vi "sub_hw-seq-all.vi"(8 "error":errorcluster, 11 "HWseq":T1) -> (0 "error out":errorcluster)   [LabVIEW 2019]
uses:
  rc-seq_enum.ctl
  SubVIs/common/_ctrl/system-status.ctl
  _ctrl/rw.ctl
  SubVIs/cmd_timer.ctl
  sequence_single.ctl
  SubVIs/common/hw-control.ctl
  common/UI.ctl
  common/cmd_timecheck.ctl
  _ctrl/BP4610_cmd.ctl
  breakdown.ctl
  SubVIs/common/cmd_offtimecheck.ctl
  _ctrl/init-r-stop.ctl
  58aef34a-c39e-4a76-bc91-cdbe2ad7e567.vi
  310223a1-0247-4d5e-a4de-31e905c381c2.vi
  d9d656a3-d7bb-48da-8160-e06b142862e8.vi
  66709171-801d-4df5-8281-070cbfffc908.vi
  b680e723-f219-401b-b6b8-117c4d919767.vi
  acb3f5d6-e9ea-41c1-b59f-33d80ec98a9a.vi
  88b04c44-2d0f-4c5f-adc0-824f85c1baca.vi
  7df0aa0f-9000-4fc8-8be1-235500cee508.vi
  a3ee31cb-2ee6-4b2e-876a-aa05c6fd3f6c.vi
  a1681bb8-cff8-4085-a791-91921f38d214.vi
  0886c58b-0a1e-4b1c-982a-d26cf992a476.vi
  1d089e96-dcf8-4fa6-b139-0f624cb7beb8.vi
  05f56422-7d15-472a-846f-8a5a9856abb2.vi
  7e616775-0fa7-4587-9f3e-cf6cd70ddc46.vi
  c0c5eac8-8ea9-47a8-809d-3af25785a4f7.vi
  9bb39240-68e1-431b-a926-99d42a230205.vi
  e7f2ea11-fc70-48eb-a069-d8d263784f6c.vi
  1f2546c3-2858-4bb2-b627-ba606493a871.vi
  SubVIs/common/Glob_Ref.vi
panel:
  in  "Numeric":i32
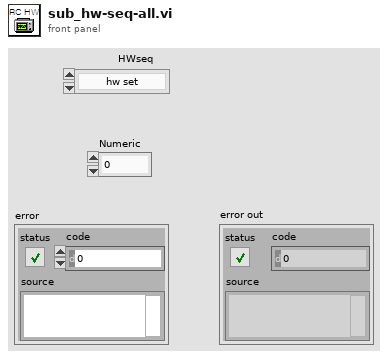
[diagram p1: front panel]
types:
  T1 = typedef "rc-seq_enum.ctl" = enum16{"hw set", "Pwr-in on", "ch-relay on", "Pwr-out on", "AO on", "AO 0v", "Pwr-in off", "Relay-all off", "Pwr-out off", "Discharge", "950 read", "Run", "Stop"}
  T2 = typedef "sequence_single.ctl" = enum16{"Register", "RC", "B1", "B2", "B3", "Oper_LV", "Oper_HV", "ContR_LV"}
  T3 = typedef "cmd_timer.ctl" = enum16{"init", "init_update", "run", "default", "update"}
  T4 = typedef "rw.ctl" = enum16{"read", "write"}
  T5 = typedef "system-status.ctl" = enum16{"Initial", "Update", "Clear", "Read"}
  T6 = typedef "ui_dev-operator.ctl" = cluster{"Operation stutus":refnum<vi>, "Test Status":refnum<vi>, "Setting":refnum<vi>, "Manual":refnum<vi>, "Main":refnum<vi>, "RCstart":refnum<vi>, "채널선택":refnum<vi>, "시험명":refnum<vi>, "Tab Control_manual":refnum<vi>, "시험 모드":refnum<vi>, "HW check":refnum<vi>, "login":refnum<vi>, "logout":refnum<vi>}
  T7 = typedef "Testing-info.ctl" = cluster{"전체채널수":u8, "현재채널번호":u8, "Irms":dbl, "입력전압":dbl, "입력전류":dbl, "출력전압":dbl, "출력전류":dbl, "온도":dbl, "제어단 단선":bool, "제어단 단락":bool, "제어단 특성변화":bool, "출력단 단선":bool, "출력단 단락":bool, "출력단 특성변화":bool, "출력단 전압":bool, "카운트 일치":bool, "Irms 판정":bool, "온도":bool, "테스트 회수":u32, "TestType":T2, "현재회수":u32, "Ch selection":cluster{"1ch":bool, "2ch":bool, "3ch":bool, "4ch":bool, "5ch":bool, "6ch":bool}, "반복":u32, "Path":path, "파일생성주기":u32, "start time":dbl, "stop time":dbl, "현재반복회수":u32, "NG":cluster{"입출력 카운트":bool, "출력전류RMS":bool}}
  T8 = cluster{"1ch":bool, "2ch":bool, "3ch":bool, "4ch":bool, "5ch":bool, "6ch":bool}
  T9 = typedef "hw-control.ctl" = enum16{"DL950 ready", "DL950 clear", "DL950 trigger", "DL950 read", "DL950 read seq", "DL950 Tsingle query", "AO 12v", "AO wave", "AO 0v", "relay all-off", "Discharge check", "Discharge", "Relay1", "Relay2", "Relay3", "Relay4", "Relay5", "Relay6", "BP4610 onoff", "BP4610 set", "DSP1500 set", "DSP1500 onoff"}
  T10 = typedef "UI.ctl" = enum16{"Alarm yellow", "DL950 graph show", "DL950 graph clear", "AO value", "AO blink onoff", "Discharge relay", "Input Power", "Outpower", "Relay in1", "Relay in2", "Relay in3", "Relay in4", "Relay in5", "Relay in6", "Relay out1", "Relay out2", "Relay out3", "Relay out4", "Relay out5", "Relay out6", "Relay all off"}
  T11 = typedef "cmd_timecheck.ctl" = enum16{"Group start", "Group end", "Grout dt", "Ch start", "Ch end", "Ch dt", "init", "NF start", "NF stop", "idrc start", "idrc stop", "scope start", "scope stop", "ao start", "ao stop", "relay start", "relay stop", "NF read start", "NF read stop", "NF set start", "NF set stop", "idrc level start", "idrc level stop", "scope trig start", "scope trig stop", "relay dischar star", "relay dischar stop", "data process start", "data process stop", "ch-relay on start", "ch-relay on stop", "hw set start", "hw set stop", "pwr-in on start", "pwr-in on stop", "pwr-out on start", "pwr-out on stop", "ao on start", "ao on stop", "ao 0v start", "ao 0v stop", "pwr-in off start", "pwr-in off stop", "relay-all off start", "relay-all off stop", "pwr-out off start", "pwr-out off stop", "discharge start", "discharge stop", "950 read start", "950 read stop"}
  T12 = typedef "BP4610_cmd.ctl" = enum16{"open", "read", "set", "set_seq", "limit", "limit_seq", "output on", "output off", "close"}
  T13 = typedef "breakdown.ctl" = enum16{"DL950 items", "input pwr", "output pwr", "output pwr_adv"}
  T14 = typedef "cmd_offtimecheck.ctl" = enum16{"start", "check", "init"}
  T15 = typedef "Error list.ctl" = cluster{"DL950":bool, "BP4610":bool, "DSP":bool, "AI":bool, "AO":bool, "DO":bool}
  T16 = typedef "init-r-stop.ctl" = enum16{"ini", "read", "stop"}
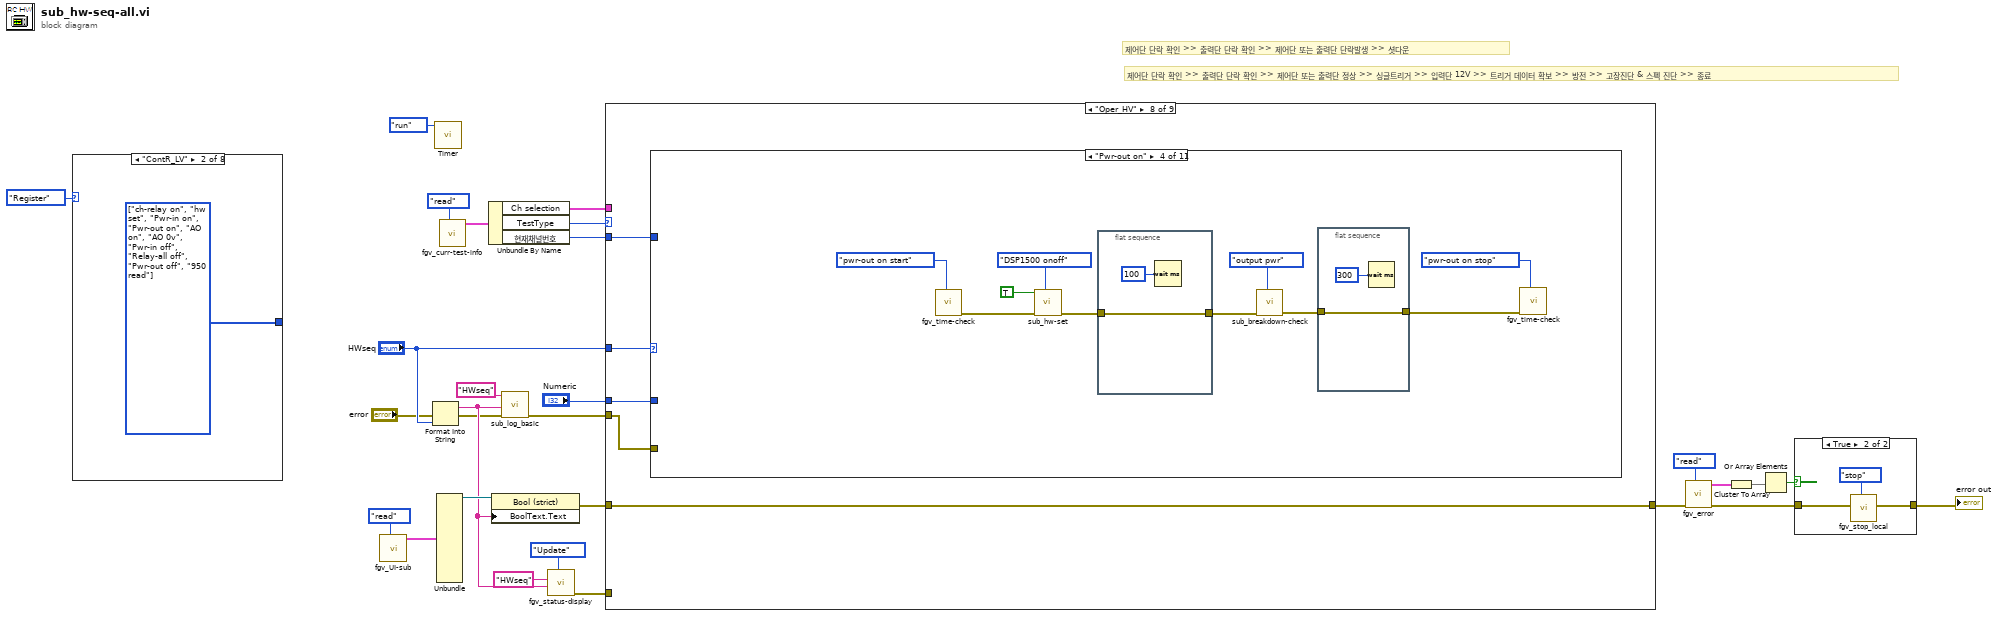
[diagram p0: block diagram]
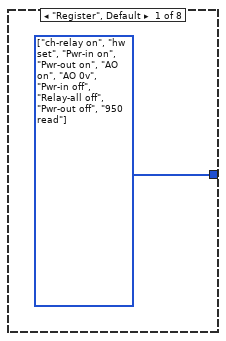
[diagram p2: hidden frame]
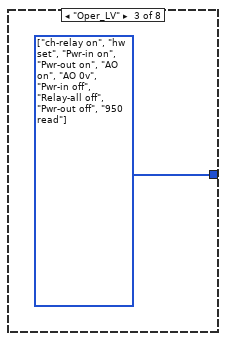
[diagram p3: hidden frame]
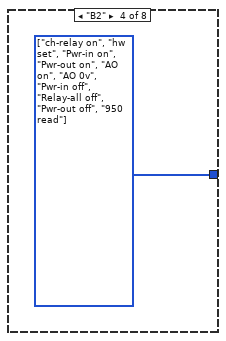
[diagram p4: hidden frame]
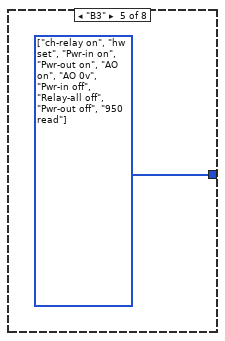
[diagram p5: hidden frame]
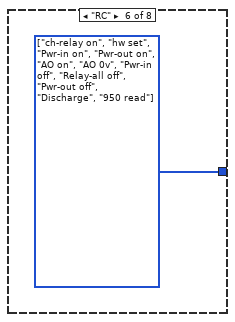
[diagram p6: hidden frame]
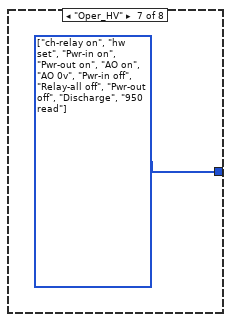
[diagram p7: hidden frame]
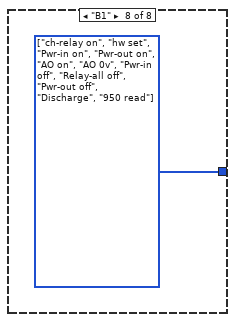
[diagram p8: hidden frame]
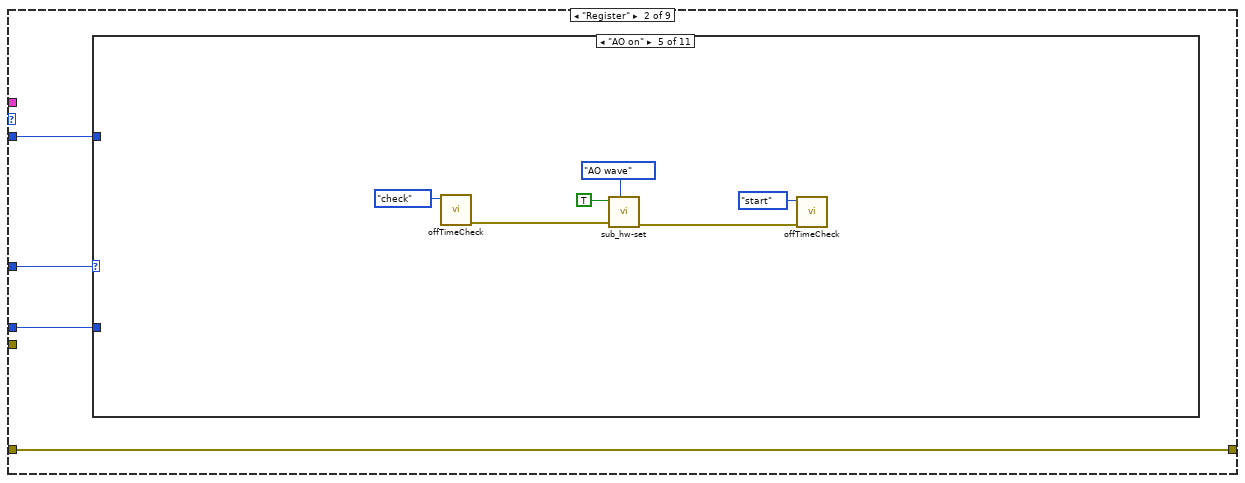
[diagram p11: hidden frame]
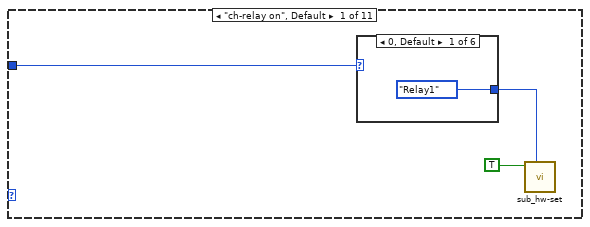
[diagram p12: hidden frame]
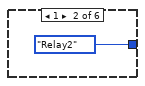
[diagram p13: hidden frame]
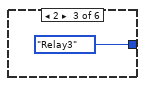
[diagram p14: hidden frame]
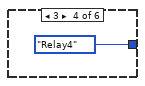
[diagram p15: hidden frame]
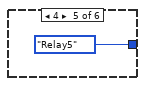
[diagram p16: hidden frame]
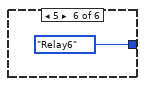
[diagram p17: hidden frame]
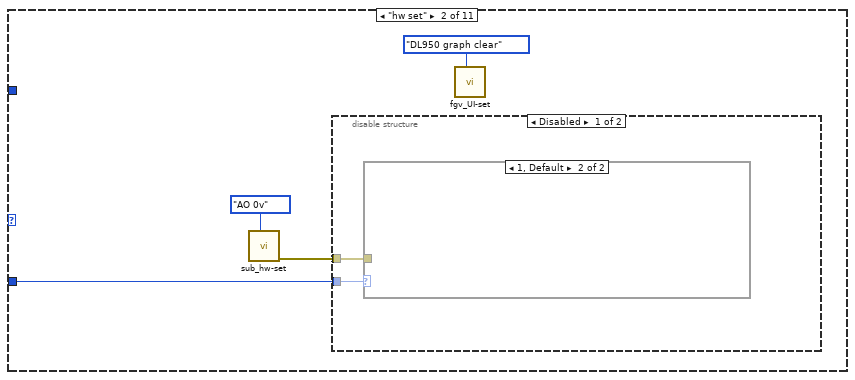
[diagram p18: hidden frame]
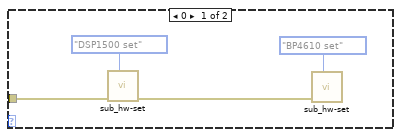
[diagram p19: hidden frame]
diagram:
  # "제어단 단락 확인 >> 출력단 단락 확인 >> 제어단 또는 출력단 정상 >> 싱글트리거 >> 입력단 12V >> 트리거 데이터 확보 >> 방전 >> 고장진단 & 스펙 진단 >> 종료"
  # "제어단 단락 확인 >> 출력단 단락 확인 >> 제어단 또는 출력단 단락발생 >> 셧다운"
  n1 = case shown="\"ContR_LV\"" sequence_single."Register" ("TestType") {
    tunnel: [w29 w30 w31 w32 w33 w34 w35 w36] -> _
    frame "Register", Default {
      w29 = T1[] [enum."ch-relay on", enum."hw set", enum."Pwr-in on", enum."Pwr-out on", enum."AO on", enum."AO 0v", enum."Pwr-in off", enum."Relay-all off", enum."Pwr-out off", enum."950 read"] items=["hw set", "Pwr-in on", "ch-relay on", "Pwr-out on", "AO on", "AO 0v", "Pwr-in off", "Relay-all off", "Pwr-out off", "Discharge", "950 read", "Run", "Stop"]
    }
    frame "ContR_LV" {
      w30 = T1[] [enum."ch-relay on", enum."hw set", enum."Pwr-in on", enum."Pwr-out on", enum."AO on", enum."AO 0v", enum."Pwr-in off", enum."Relay-all off", enum."Pwr-out off", enum."950 read"] items=["hw set", "Pwr-in on", "ch-relay on", "Pwr-out on", "AO on", "AO 0v", "Pwr-in off", "Relay-all off", "Pwr-out off", "Discharge", "950 read", "Run", "Stop"]
    }
    frame "Oper_LV" {
      w31 = T1[] [enum."ch-relay on", enum."hw set", enum."Pwr-in on", enum."Pwr-out on", enum."AO on", enum."AO 0v", enum."Pwr-in off", enum."Relay-all off", enum."Pwr-out off", enum."950 read"] items=["hw set", "Pwr-in on", "ch-relay on", "Pwr-out on", "AO on", "AO 0v", "Pwr-in off", "Relay-all off", "Pwr-out off", "Discharge", "950 read", "Run", "Stop"]
    }
    frame "B2" {
      w32 = T1[] [enum."ch-relay on", enum."hw set", enum."Pwr-in on", enum."Pwr-out on", enum."AO on", enum."AO 0v", enum."Pwr-in off", enum."Relay-all off", enum."Pwr-out off", enum."950 read"] items=["hw set", "Pwr-in on", "ch-relay on", "Pwr-out on", "AO on", "AO 0v", "Pwr-in off", "Relay-all off", "Pwr-out off", "Discharge", "950 read", "Run", "Stop"]
    }
    frame "B3" {
      w33 = T1[] [enum."ch-relay on", enum."hw set", enum."Pwr-in on", enum."Pwr-out on", enum."AO on", enum."AO 0v", enum."Pwr-in off", enum."Relay-all off", enum."Pwr-out off", enum."950 read"] items=["hw set", "Pwr-in on", "ch-relay on", "Pwr-out on", "AO on", "AO 0v", "Pwr-in off", "Relay-all off", "Pwr-out off", "Discharge", "950 read", "Run", "Stop"]
    }
    frame "RC" {
      w34 = T1[] [enum."ch-relay on", enum."hw set", enum."Pwr-in on", enum."Pwr-out on", enum."AO on", enum."AO 0v", enum."Pwr-in off", enum."Relay-all off", enum."Pwr-out off", enum."Discharge", enum."950 read"] items=["hw set", "Pwr-in on", "ch-relay on", "Pwr-out on", "AO on", "AO 0v", "Pwr-in off", "Relay-all off", "Pwr-out off", "Discharge", "950 read", "Run", "Stop"]
    }
    frame "Oper_HV" {
      w35 = T1[] [enum."ch-relay on", enum."hw set", enum."Pwr-in on", enum."Pwr-out on", enum."AO on", enum."AO 0v", enum."Pwr-in off", enum."Relay-all off", enum."Pwr-out off", enum."Discharge", enum."950 read"] items=["hw set", "Pwr-in on", "ch-relay on", "Pwr-out on", "AO on", "AO 0v", "Pwr-in off", "Relay-all off", "Pwr-out off", "Discharge", "950 read", "Run", "Stop"]
    }
    frame "B1" {
      w36 = T1[] [enum."ch-relay on", enum."hw set", enum."Pwr-in on", enum."Pwr-out on", enum."AO on", enum."AO 0v", enum."Pwr-in off", enum."Relay-all off", enum."Pwr-out off", enum."Discharge", enum."950 read"] items=["hw set", "Pwr-in on", "ch-relay on", "Pwr-out on", "AO on", "AO 0v", "Pwr-in off", "Relay-all off", "Pwr-out off", "Discharge", "950 read", "Run", "Stop"]
    }
  }
  n2 = call "fgv_UI-sub.vi"("cmd"=rw."read") -> ("output cluster 2"=w22:T6)  [unwired: 9 in, 1 out]
  n3 = Format Into String(error in="error", "HWseq") -> (resulting string=w17:string, error out=w3:errorcluster)  [unwired: 2 in]
  n4 = call "Timer.vi"("cmd"=cmd_timer."run") -> ()  [unwired: 8 in, 3 out]
  n5 = Unbundle(w22) -> ("Operation stutus"=w21:refnum<vi>)  [unwired: 12 out]
  n6 = call "fgv_curr-test-info.vi"("cmd"=rw."read") -> ("현재테스트 정보 2"=w28:T7)  [unwired: 10 in]
  n7 = Unbundle By Name(w28) -> ("Ch selection"=w26:T8, "TestType"=w25:T2, "현재채널번호"=w13:u8)
  n8 = property class="Bool (strict)"(reference=w21, "BoolText.Text"=w17) -> (error out=w15:errorcluster)  [unwired: 1 in, 1 out]
  n9 = call "sub_log_basic.vi"("error in"=w3, "desc"=w17, "Title"="HWseq") -> ("error out"=w14:errorcluster)  [unwired: 8 in]
  n10 = call "fgv_status-display.vi"("Mode"=system-status."Update", "detail"=w17, "title"="HWseq") -> ("error out"=w16:errorcluster)  [unwired: 8 in]
  n11 = case shown="\"Oper_HV\"" w25 {
    tunnel: w13 -> [_ w41 w148 w254 w359 w465 w570 w680 w787]
    tunnel: "HWseq" -> [_ w40 w147 w253 w358 w464 w569 w679 w786]
    tunnel: w26 -> [_ _ _ _ _ _ _ _ _]
    tunnel: w16 -> [_ _ _ _ _ _ _ _ _]
    tunnel: w15 -> [w37 w38 w144 w250 w356 w462 w567 w676 w784]
    tunnel: w14 -> [_ _ w145 w251 _ _ _ w677 _]
    tunnel: "Numeric" -> [_ w39 w146 w252 w357 w463 w568 w678 w785]
    tunnel: [w37 w38 w144 w250 w356 w462 w567 w676 w784] -> w9
    frame Default {
    }
    frame "Register" {
      n12 = case shown="\"AO on\"" w40 {
        tunnel: w41 -> [w42 _ _ _ _ _ _ _ _ _ w143]
        tunnel: w39 -> [_ w51 _ _ _ _ _ _ _ _ _]
        frame "ch-relay on", Default {
          n13 = case shown="0, Default" w42 {
            tunnel: [hw-control."Relay1" ("cmd") hw-control."Relay2" ("cmd") hw-control."Relay3" ("cmd") hw-control."Relay4" ("cmd") hw-control."Relay5" ("cmd") hw-control."Relay6" ("cmd")] -> w43
            frame 0, Default {
            }
            frame 1 {
            }
            frame 2 {
            }
            frame 3 {
            }
            frame 4 {
            }
            frame 5 {
            }
          }
          n14 = call "sub_hw-set.vi"("cmd"=w43, "onoff"=TRUE) -> ()  [unwired: 9 in, 1 out]
        }
        frame "hw set" {
          n15 = call "sub_hw-set.vi"("cmd"=hw-control."AO 0v") -> ("error out"=w52:errorcluster)  [unwired: 10 in]
          n16 = disable-structure shown="Disabled" {
            disable-tunnel: w52 -> [w56 _]
            disable-tunnel: w51 -> [w55 _]
            frame Disabled {
              n17 = case shown="1, Default" w55 {
                tunnel: w56 -> [w58 _]
                frame 0 {
                  n18 = call "sub_hw-set.vi"("cmd"=hw-control."DSP1500 set", "error in"=w58) -> ("error out"=w57:errorcluster)  [unwired: 9 in]
                  n19 = call "sub_hw-set.vi"("cmd"=hw-control."BP4610 set", "error in"=w57) -> ()  [unwired: 9 in, 1 out]
                }
                frame 1, Default {
                }
              }
            }
            frame Enabled {
            }
          }
          n20 = call "fgv_UI-set.vi"("cmd"=UI."DL950 graph clear") -> ()  [unwired: 10 in, 1 out]
        }
        frame "Pwr-in on" {
          n21 = call "fgv_time-check.vi"("cmd"=cmd_timecheck."pwr-in on start") -> ("error out"=w65:errorcluster)  [unwired: 9 in, 1 out]
          n22 = call "sub_hw-set.vi"("cmd"=hw-control."BP4610 onoff", "error in"=w65, "onoff"=TRUE) -> ("error out"=w64:errorcluster)  [unwired: 8 in]
          n23 = call "sub_hw-set.vi"("cmd"=hw-control."AO 12v", "error in"=w64) -> ("error out"=w63:errorcluster)  [unwired: 9 in]
          n24 = Wait (ms)(milliseconds to wait=u32 100) -> ()  [unwired: 1 out]
          n25 = call "Stall Data Flow.vim"("value in"=w63, "milliseconds to wait"=u32 500 ("dt")) -> ("value out"=w72:errorcluster)  [unwired: 1 out]
          n26 = call "fgv_time-check.vi"("cmd"=cmd_timecheck."NF read start", "error in (no error)"=w72) -> ("error out"=w71:errorcluster)  [unwired: 8 in, 1 out]
          n27 = for {
            N: 3 -> [_]
            shift-right: [w82] -> w69
            shift-left: w71 -> [w83]
            n28 = call "fgv_4610_visa.vi"("cmd"=BP4610_cmd."read", "error in"=w83) -> ("error out"=w82:errorcluster)  [unwired: 9 in]
          }
          n29 = call "fgv_time-check.vi"("cmd"=cmd_timecheck."NF read stop", "error in (no error)"=w69) -> ("error out"=w68:errorcluster)  [unwired: 8 in, 1 out]
          n30 = call "Stall Data Flow.vim"("value in"=w68, "milliseconds to wait"=u32 200 ("dt")) -> ("value out"=w62:errorcluster)  [unwired: 1 out]
          n31 = call "sub_hw-set.vi"("cmd"=hw-control."AO 0v", "error in"=w62) -> ("error out"=w61:errorcluster)  [unwired: 9 in]
          n32 = call "fgv_time-check.vi"("cmd"=cmd_timecheck."pwr-in on stop", "error in (no error)"=w61) -> ()  [unwired: 8 in, 2 out]
        }
        frame "Pwr-out on" {
          n33 = call "fgv_time-check.vi"("cmd"=cmd_timecheck."pwr-out on start") -> ("error out"=w87:errorcluster)  [unwired: 9 in, 1 out]
          n34 = call "sub_hw-set.vi"("cmd"=hw-control."DSP1500 onoff", "error in"=w87, "onoff"=TRUE) -> ("error out"=w90:errorcluster)  [unwired: 8 in]
          n35 = flat-sequence {
            tunnel: [w97] -> w91
            tunnel: w90 -> [w97]
            frame #0 {
              n36 = Wait (ms)(milliseconds to wait=u32 200) -> ()  [unwired: 1 out]
            }
          }
          n37 = call "sub_breakdown-check.vi"("breakdown type"=breakdown."output pwr", "error in (no error)"=w91) -> ("error out"=w89:errorcluster)  [unwired: 9 in]
          n38 = flat-sequence {
            tunnel: w89 -> [w95]
            tunnel: [w95] -> w85
            frame #0 {
              n39 = Wait (ms)(milliseconds to wait=u32 500) -> ()  [unwired: 1 out]
            }
          }
          n40 = call "fgv_time-check.vi"("cmd"=cmd_timecheck."pwr-out on stop", "error in (no error)"=w85) -> ()  [unwired: 8 in, 2 out]
        }
        frame "AO on" {
          n41 = call "offTimeCheck.vi"("cmd"=cmd_offtimecheck."check") -> ("error out"=w100:errorcluster)  [unwired: 10 in]
          n42 = call "sub_hw-set.vi"("cmd"=hw-control."AO wave", "error in"=w100, "onoff"=TRUE) -> ("error out"=w99:errorcluster)  [unwired: 8 in]
          n43 = call "offTimeCheck.vi"("error in (no error)"=w99, "cmd"=cmd_offtimecheck."start") -> ()  [unwired: 9 in, 1 out]
        }
        frame "AO 0v" {
          n44 = disable-structure shown="Disabled" {
            frame Disabled {
              n45 = call "sub_hw-set.vi"("cmd"=hw-control."AO 0v") -> ()  [unwired: 10 in, 1 out]
            }
            frame Enabled {
            }
          }
        }
        frame "Pwr-in off" {
          n46 = call "fgv_time-check.vi"("cmd"=cmd_timecheck."pwr-in off start") -> ("error out"=w108:errorcluster)  [unwired: 9 in, 1 out]
          n47 = call "sub_hw-set.vi"("cmd"=hw-control."BP4610 onoff", "error in"=w108, "onoff"=FALSE) -> ("error out"=w106:errorcluster)  [unwired: 8 in]
          n48 = call "fgv_time-check.vi"("cmd"=cmd_timecheck."pwr-in off start", "error in (no error)"=w106) -> ()  [unwired: 8 in, 2 out]
        }
        frame "Relay-all off" {
          n49 = call "fgv_time-check.vi"("cmd"=cmd_timecheck."relay-all off start") -> ("error out"=w114:errorcluster)  [unwired: 9 in, 1 out]
          n50 = call "sub_hw-set.vi"("cmd"=hw-control."relay all-off", "error in"=w114, "onoff"=FALSE) -> ("error out"=w112:errorcluster)  [unwired: 8 in]
          n51 = call "fgv_time-check.vi"("cmd"=cmd_timecheck."relay-all off stop", "error in (no error)"=w112) -> ()  [unwired: 8 in, 2 out]
        }
        frame "Pwr-out off" {
          n52 = call "fgv_time-check.vi"("cmd"=cmd_timecheck."pwr-out off start") -> ("error out"=w120:errorcluster)  [unwired: 9 in, 1 out]
          n53 = call "sub_hw-set.vi"("cmd"=hw-control."DSP1500 onoff", "error in"=w120, "onoff"=FALSE) -> ("error out"=w118:errorcluster)  [unwired: 8 in]
          n54 = call "fgv_time-check.vi"("cmd"=cmd_timecheck."pwr-out off stop", "error in (no error)"=w118) -> ()  [unwired: 8 in, 2 out]
        }
        frame "Discharge" {
          n55 = call "fgv_time-check.vi"("cmd"=cmd_timecheck."discharge start") -> ("error out"=w129:errorcluster)  [unwired: 9 in, 1 out]
          n56 = call "sub_hw-set.vi"("cmd"=hw-control."Discharge", "error in"=w129, "onoff"=TRUE) -> ("error out"=w128:errorcluster)  [unwired: 8 in]
          n57 = call "sub_hw-set.vi"("cmd"=hw-control."Discharge check", "error in"=w128) -> ("error out"=w127:errorcluster)  [unwired: 9 in]
          n58 = call "sub_hw-set.vi"("cmd"=hw-control."Discharge", "error in"=w127, "onoff"=FALSE) -> ("error out"=w124:errorcluster)  [unwired: 8 in]
          n59 = flat-sequence {
            tunnel: [w136] -> w125
            tunnel: w124 -> [w136]
            frame #0 {
              n60 = Wait (ms)(milliseconds to wait=u32 2000) -> ()  [unwired: 1 out]
            }
          }
          n61 = call "fgv_time-check.vi"("cmd"=cmd_timecheck."discharge stop", "error in (no error)"=w125) -> ()  [unwired: 8 in, 2 out]
        }
        frame "950 read" {
          n62 = call "fgv_time-check.vi"("cmd"=cmd_timecheck."950 read start") -> ("error out"=w140:errorcluster)  [unwired: 9 in, 1 out]
          n63 = call "sub_hw-set.vi"("cmd"=hw-control."DL950 read seq", "error in"=w140, "DUT Ch"=w143) -> ("error out"=w138:errorcluster)  [unwired: 8 in]
          n64 = call "fgv_time-check.vi"("cmd"=cmd_timecheck."950 read stop", "error in (no error)"=w138) -> ()  [unwired: 8 in, 2 out]
        }
      }
    }
    frame "RC" {
      n65 = case shown="\"AO on\"" w147 {
        tunnel: w145 -> [_ _ _ _ _ _ _ _ _ _ _]
        tunnel: w148 -> [w149 _ _ _ _ _ _ _ _ _ w249]
        tunnel: w146 -> [_ w158 _ _ _ _ _ _ _ _ _]
        frame "ch-relay on", Default {
          n66 = case shown="0, Default" w149 {
            tunnel: [hw-control."Relay1" ("cmd") hw-control."Relay2" ("cmd") hw-control."Relay3" ("cmd") hw-control."Relay4" ("cmd") hw-control."Relay5" ("cmd") hw-control."Relay6" ("cmd")] -> w150
            frame 0, Default {
            }
            frame 1 {
            }
            frame 2 {
            }
            frame 3 {
            }
            frame 4 {
            }
            frame 5 {
            }
          }
          n67 = call "sub_hw-set.vi"("cmd"=w150, "onoff"=TRUE) -> ()  [unwired: 9 in, 1 out]
        }
        frame "hw set" {
          n68 = call "sub_hw-set.vi"("cmd"=hw-control."AO 0v") -> ("error out"=w159:errorcluster)  [unwired: 10 in]
          n69 = disable-structure shown="Disabled" {
            disable-tunnel: w159 -> [w163 _]
            disable-tunnel: w158 -> [w162 _]
            frame Disabled {
              n70 = case shown="1, Default" w162 {
                tunnel: w163 -> [w165 _]
                frame 0 {
                  n71 = call "sub_hw-set.vi"("cmd"=hw-control."DSP1500 set", "error in"=w165) -> ("error out"=w164:errorcluster)  [unwired: 9 in]
                  n72 = call "sub_hw-set.vi"("cmd"=hw-control."BP4610 set", "error in"=w164) -> ()  [unwired: 9 in, 1 out]
                }
                frame 1, Default {
                }
              }
              n73 = call "fgv_UI-set.vi"("cmd"=UI."DL950 graph clear") -> ()  [unwired: 10 in, 1 out]
            }
            frame Enabled {
            }
          }
        }
        frame "Pwr-in on" {
          n74 = call "fgv_time-check.vi"("cmd"=cmd_timecheck."pwr-in on start") -> ("error out"=w172:errorcluster)  [unwired: 9 in, 1 out]
          n75 = call "sub_hw-set.vi"("cmd"=hw-control."BP4610 onoff", "error in"=w172, "onoff"=TRUE) -> ("error out"=w171:errorcluster)  [unwired: 8 in]
          n76 = call "sub_hw-set.vi"("cmd"=hw-control."AO 12v", "error in"=w171) -> ("error out"=w170:errorcluster)  [unwired: 9 in]
          n77 = call "Stall Data Flow.vim"("value in"=w170, "milliseconds to wait"=u32 200 ("dt")) -> ("value out"=w179:errorcluster)  [unwired: 1 out]
          n78 = call "fgv_time-check.vi"("cmd"=cmd_timecheck."NF read start", "error in (no error)"=w179) -> ("error out"=w178:errorcluster)  [unwired: 8 in, 1 out]
          n79 = for {
            N: 3 -> [_]
            shift-right: [w188] -> w176
            shift-left: w178 -> [w189]
            n80 = call "fgv_4610_visa.vi"("cmd"=BP4610_cmd."read", "error in"=w189) -> ("error out"=w188:errorcluster)  [unwired: 9 in]
          }
          n81 = call "fgv_time-check.vi"("cmd"=cmd_timecheck."NF read stop", "error in (no error)"=w176) -> ("error out"=w175:errorcluster)  [unwired: 8 in, 1 out]
          n82 = call "Stall Data Flow.vim"("value in"=w175, "milliseconds to wait"=u32 200 ("dt")) -> ("value out"=w169:errorcluster)  [unwired: 1 out]
          n83 = call "sub_hw-set.vi"("cmd"=hw-control."AO 0v", "error in"=w169) -> ("error out"=w168:errorcluster)  [unwired: 9 in]
          n84 = call "fgv_time-check.vi"("cmd"=cmd_timecheck."pwr-in on stop", "error in (no error)"=w168) -> ()  [unwired: 8 in, 2 out]
        }
        frame "Pwr-out on" {
          n85 = call "fgv_time-check.vi"("cmd"=cmd_timecheck."pwr-out on start") -> ("error out"=w193:errorcluster)  [unwired: 9 in, 1 out]
          n86 = call "sub_hw-set.vi"("cmd"=hw-control."DSP1500 onoff", "error in"=w193, "onoff"=TRUE) -> ("error out"=w196:errorcluster)  [unwired: 8 in]
          n87 = flat-sequence {
            tunnel: [w203] -> w197
            tunnel: w196 -> [w203]
            frame #0 {
              n88 = Wait (ms)(milliseconds to wait=u32 100) -> ()  [unwired: 1 out]
            }
          }
          n89 = call "sub_breakdown-check.vi"("breakdown type"=breakdown."output pwr", "error in (no error)"=w197) -> ("error out"=w195:errorcluster)  [unwired: 9 in]
          n90 = flat-sequence {
            tunnel: w195 -> [w201]
            tunnel: [w201] -> w191
            frame #0 {
              n91 = Wait (ms)(milliseconds to wait=u32 400) -> ()  [unwired: 1 out]
            }
          }
          n92 = call "fgv_time-check.vi"("cmd"=cmd_timecheck."pwr-out on stop", "error in (no error)"=w191) -> ()  [unwired: 8 in, 2 out]
        }
        frame "AO on" {
          n93 = call "offTimeCheck.vi"("cmd"=cmd_offtimecheck."check") -> ("error out"=w206:errorcluster)  [unwired: 10 in]
          n94 = call "sub_hw-set.vi"("cmd"=hw-control."AO wave", "error in"=w206, "onoff"=TRUE) -> ("error out"=w205:errorcluster)  [unwired: 8 in]
          n95 = call "offTimeCheck.vi"("error in (no error)"=w205, "cmd"=cmd_offtimecheck."start") -> ()  [unwired: 9 in, 1 out]
        }
        frame "AO 0v" {
          n96 = disable-structure shown="Disabled" {
            frame Disabled {
              n97 = call "sub_hw-set.vi"("cmd"=hw-control."AO 0v") -> ()  [unwired: 10 in, 1 out]
            }
            frame Enabled {
            }
          }
        }
        frame "Pwr-in off" {
          n98 = call "fgv_time-check.vi"("cmd"=cmd_timecheck."pwr-in off start") -> ("error out"=w214:errorcluster)  [unwired: 9 in, 1 out]
          n99 = call "sub_hw-set.vi"("cmd"=hw-control."BP4610 onoff", "error in"=w214, "onoff"=FALSE) -> ("error out"=w212:errorcluster)  [unwired: 8 in]
          n100 = call "fgv_time-check.vi"("cmd"=cmd_timecheck."pwr-in off start", "error in (no error)"=w212) -> ()  [unwired: 8 in, 2 out]
        }
        frame "Relay-all off" {
          n101 = call "fgv_time-check.vi"("cmd"=cmd_timecheck."relay-all off start") -> ("error out"=w220:errorcluster)  [unwired: 9 in, 1 out]
          n102 = call "sub_hw-set.vi"("cmd"=hw-control."relay all-off", "error in"=w220, "onoff"=FALSE) -> ("error out"=w218:errorcluster)  [unwired: 8 in]
          n103 = call "fgv_time-check.vi"("cmd"=cmd_timecheck."relay-all off stop", "error in (no error)"=w218) -> ()  [unwired: 8 in, 2 out]
        }
        frame "Pwr-out off" {
          n104 = call "fgv_time-check.vi"("cmd"=cmd_timecheck."pwr-out off start") -> ("error out"=w226:errorcluster)  [unwired: 9 in, 1 out]
          n105 = call "sub_hw-set.vi"("cmd"=hw-control."DSP1500 onoff", "error in"=w226, "onoff"=FALSE) -> ("error out"=w224:errorcluster)  [unwired: 8 in]
          n106 = call "fgv_time-check.vi"("cmd"=cmd_timecheck."pwr-out off stop", "error in (no error)"=w224) -> ()  [unwired: 8 in, 2 out]
        }
        frame "Discharge" {
          n107 = call "fgv_time-check.vi"("cmd"=cmd_timecheck."discharge start") -> ("error out"=w235:errorcluster)  [unwired: 9 in, 1 out]
          n108 = call "sub_hw-set.vi"("cmd"=hw-control."Discharge", "error in"=w235, "onoff"=TRUE) -> ("error out"=w234:errorcluster)  [unwired: 8 in]
          n109 = call "sub_hw-set.vi"("cmd"=hw-control."Discharge check", "error in"=w234) -> ("error out"=w233:errorcluster)  [unwired: 9 in]
          n110 = call "sub_hw-set.vi"("cmd"=hw-control."Discharge", "error in"=w233, "onoff"=FALSE) -> ("error out"=w230:errorcluster)  [unwired: 8 in]
          n111 = flat-sequence {
            tunnel: [w242] -> w231
            tunnel: w230 -> [w242]
            frame #0 {
              n112 = Wait (ms)(milliseconds to wait=u32 2000) -> ()  [unwired: 1 out]
            }
          }
          n113 = call "fgv_time-check.vi"("cmd"=cmd_timecheck."discharge stop", "error in (no error)"=w231) -> ()  [unwired: 8 in, 2 out]
        }
        frame "950 read" {
          n114 = call "fgv_time-check.vi"("cmd"=cmd_timecheck."950 read start") -> ("error out"=w246:errorcluster)  [unwired: 9 in, 1 out]
          n115 = call "sub_hw-set.vi"("cmd"=hw-control."DL950 read seq", "error in"=w246, "DUT Ch"=w249) -> ("error out"=w244:errorcluster)  [unwired: 8 in]
          n116 = call "fgv_time-check.vi"("cmd"=cmd_timecheck."950 read stop", "error in (no error)"=w244) -> ()  [unwired: 8 in, 2 out]
        }
      }
    }
    frame "B1" {
      n117 = case shown="\"AO on\"" w253 {
        tunnel: w251 -> [_ _ _ _ _ _ _ _ _ _ _]
        tunnel: w254 -> [w255 _ _ _ _ _ _ _ _ _ w355]
        tunnel: w252 -> [_ w264 _ _ _ _ _ _ _ _ _]
        frame "ch-relay on", Default {
          n118 = case shown="0, Default" w255 {
            tunnel: [hw-control."Relay1" ("cmd") hw-control."Relay2" ("cmd") hw-control."Relay3" ("cmd") hw-control."Relay4" ("cmd") hw-control."Relay5" ("cmd") hw-control."Relay6" ("cmd")] -> w256
            frame 0, Default {
            }
            frame 1 {
            }
            frame 2 {
            }
            frame 3 {
            }
            frame 4 {
            }
            frame 5 {
            }
          }
          n119 = call "sub_hw-set.vi"("cmd"=w256, "onoff"=TRUE) -> ()  [unwired: 9 in, 1 out]
        }
        frame "hw set" {
          n120 = call "sub_hw-set.vi"("cmd"=hw-control."AO 0v") -> ("error out"=w265:errorcluster)  [unwired: 10 in]
          n121 = disable-structure shown="Disabled" {
            disable-tunnel: w265 -> [w269 _]
            disable-tunnel: w264 -> [w268 _]
            frame Disabled {
              n122 = case shown="1, Default" w268 {
                tunnel: w269 -> [w271 _]
                frame 0 {
                  n123 = call "sub_hw-set.vi"("cmd"=hw-control."DSP1500 set", "error in"=w271) -> ("error out"=w270:errorcluster)  [unwired: 9 in]
                  n124 = call "sub_hw-set.vi"("cmd"=hw-control."BP4610 set", "error in"=w270) -> ()  [unwired: 9 in, 1 out]
                }
                frame 1, Default {
                }
              }
              n125 = call "fgv_UI-set.vi"("cmd"=UI."DL950 graph clear") -> ()  [unwired: 10 in, 1 out]
            }
            frame Enabled {
            }
          }
        }
        frame "Pwr-in on" {
          n126 = call "fgv_time-check.vi"("cmd"=cmd_timecheck."pwr-in on start") -> ("error out"=w278:errorcluster)  [unwired: 9 in, 1 out]
          n127 = call "sub_hw-set.vi"("cmd"=hw-control."BP4610 onoff", "error in"=w278, "onoff"=TRUE) -> ("error out"=w277:errorcluster)  [unwired: 8 in]
          n128 = call "sub_hw-set.vi"("cmd"=hw-control."AO 12v", "error in"=w277) -> ("error out"=w276:errorcluster)  [unwired: 9 in]
          n129 = call "Stall Data Flow.vim"("value in"=w276, "milliseconds to wait"=u32 200 ("dt")) -> ("value out"=w285:errorcluster)  [unwired: 1 out]
          n130 = call "fgv_time-check.vi"("cmd"=cmd_timecheck."NF read start", "error in (no error)"=w285) -> ("error out"=w284:errorcluster)  [unwired: 8 in, 1 out]
          n131 = for {
            N: 3 -> [_]
            shift-right: [w294] -> w282
            shift-left: w284 -> [w295]
            n132 = call "fgv_4610_visa.vi"("cmd"=BP4610_cmd."read", "error in"=w295) -> ("error out"=w294:errorcluster)  [unwired: 9 in]
          }
          n133 = call "fgv_time-check.vi"("cmd"=cmd_timecheck."NF read stop", "error in (no error)"=w282) -> ("error out"=w281:errorcluster)  [unwired: 8 in, 1 out]
          n134 = call "Stall Data Flow.vim"("value in"=w281, "milliseconds to wait"=u32 200 ("dt")) -> ("value out"=w275:errorcluster)  [unwired: 1 out]
          n135 = call "sub_hw-set.vi"("cmd"=hw-control."AO 0v", "error in"=w275) -> ("error out"=w274:errorcluster)  [unwired: 9 in]
          n136 = call "fgv_time-check.vi"("cmd"=cmd_timecheck."pwr-in on stop", "error in (no error)"=w274) -> ()  [unwired: 8 in, 2 out]
        }
        frame "Pwr-out on" {
          n137 = call "fgv_time-check.vi"("cmd"=cmd_timecheck."pwr-out on start") -> ("error out"=w299:errorcluster)  [unwired: 9 in, 1 out]
          n138 = call "sub_hw-set.vi"("cmd"=hw-control."DSP1500 onoff", "error in"=w299, "onoff"=TRUE) -> ("error out"=w302:errorcluster)  [unwired: 8 in]
          n139 = flat-sequence {
            tunnel: [w309] -> w303
            tunnel: w302 -> [w309]
            frame #0 {
              n140 = Wait (ms)(milliseconds to wait=u32 200) -> ()  [unwired: 1 out]
            }
          }
          n141 = call "sub_breakdown-check.vi"("breakdown type"=breakdown."output pwr", "error in (no error)"=w303) -> ("error out"=w301:errorcluster)  [unwired: 9 in]
          n142 = flat-sequence {
            tunnel: w301 -> [w307]
            tunnel: [w307] -> w297
            frame #0 {
              n143 = Wait (ms)(milliseconds to wait=u32 400) -> ()  [unwired: 1 out]
            }
          }
          n144 = call "fgv_time-check.vi"("cmd"=cmd_timecheck."pwr-out on stop", "error in (no error)"=w297) -> ()  [unwired: 8 in, 2 out]
        }
        frame "AO on" {
          n145 = call "offTimeCheck.vi"("cmd"=cmd_offtimecheck."check") -> ("error out"=w312:errorcluster)  [unwired: 10 in]
          n146 = call "sub_hw-set.vi"("cmd"=hw-control."AO wave", "error in"=w312, "onoff"=TRUE) -> ("error out"=w311:errorcluster)  [unwired: 8 in]
          n147 = call "offTimeCheck.vi"("error in (no error)"=w311, "cmd"=cmd_offtimecheck."start") -> ()  [unwired: 9 in, 1 out]
        }
        frame "AO 0v" {
          n148 = disable-structure shown="Disabled" {
            frame Disabled {
              n149 = call "sub_hw-set.vi"("cmd"=hw-control."AO 0v") -> ()  [unwired: 10 in, 1 out]
            }
            frame Enabled {
            }
          }
        }
        frame "Pwr-in off" {
          n150 = call "fgv_time-check.vi"("cmd"=cmd_timecheck."pwr-in off start") -> ("error out"=w320:errorcluster)  [unwired: 9 in, 1 out]
          n151 = call "sub_hw-set.vi"("cmd"=hw-control."BP4610 onoff", "error in"=w320, "onoff"=FALSE) -> ("error out"=w318:errorcluster)  [unwired: 8 in]
          n152 = call "fgv_time-check.vi"("cmd"=cmd_timecheck."pwr-in off start", "error in (no error)"=w318) -> ()  [unwired: 8 in, 2 out]
        }
        frame "Relay-all off" {
          n153 = call "fgv_time-check.vi"("cmd"=cmd_timecheck."relay-all off start") -> ("error out"=w326:errorcluster)  [unwired: 9 in, 1 out]
          n154 = call "sub_hw-set.vi"("cmd"=hw-control."relay all-off", "error in"=w326, "onoff"=FALSE) -> ("error out"=w324:errorcluster)  [unwired: 8 in]
          n155 = call "fgv_time-check.vi"("cmd"=cmd_timecheck."relay-all off stop", "error in (no error)"=w324) -> ()  [unwired: 8 in, 2 out]
        }
        frame "Pwr-out off" {
          n156 = call "fgv_time-check.vi"("cmd"=cmd_timecheck."pwr-out off start") -> ("error out"=w332:errorcluster)  [unwired: 9 in, 1 out]
          n157 = call "sub_hw-set.vi"("cmd"=hw-control."DSP1500 onoff", "error in"=w332, "onoff"=FALSE) -> ("error out"=w330:errorcluster)  [unwired: 8 in]
          n158 = call "fgv_time-check.vi"("cmd"=cmd_timecheck."pwr-out off stop", "error in (no error)"=w330) -> ()  [unwired: 8 in, 2 out]
        }
        frame "Discharge" {
          n159 = call "fgv_time-check.vi"("cmd"=cmd_timecheck."discharge start") -> ("error out"=w341:errorcluster)  [unwired: 9 in, 1 out]
          n160 = call "sub_hw-set.vi"("cmd"=hw-control."Discharge", "error in"=w341, "onoff"=TRUE) -> ("error out"=w340:errorcluster)  [unwired: 8 in]
          n161 = call "sub_hw-set.vi"("cmd"=hw-control."Discharge check", "error in"=w340) -> ("error out"=w339:errorcluster)  [unwired: 9 in]
          n162 = call "sub_hw-set.vi"("cmd"=hw-control."Discharge", "error in"=w339, "onoff"=FALSE) -> ("error out"=w336:errorcluster)  [unwired: 8 in]
          n163 = flat-sequence {
            tunnel: [w348] -> w337
            tunnel: w336 -> [w348]
            frame #0 {
              n164 = Wait (ms)(milliseconds to wait=u32 2000) -> ()  [unwired: 1 out]
            }
          }
          n165 = call "fgv_time-check.vi"("cmd"=cmd_timecheck."discharge stop", "error in (no error)"=w337) -> ()  [unwired: 8 in, 2 out]
        }
        frame "950 read" {
          n166 = call "fgv_time-check.vi"("cmd"=cmd_timecheck."950 read start") -> ("error out"=w352:errorcluster)  [unwired: 9 in, 1 out]
          n167 = call "sub_hw-set.vi"("cmd"=hw-control."DL950 read seq", "error in"=w352, "DUT Ch"=w355) -> ("error out"=w350:errorcluster)  [unwired: 8 in]
          n168 = call "fgv_time-check.vi"("cmd"=cmd_timecheck."950 read stop", "error in (no error)"=w350) -> ()  [unwired: 8 in, 2 out]
        }
      }
    }
    frame "B2" {
      n169 = case shown="\"AO on\"" w358 {
        tunnel: w359 -> [w360 _ _ _ _ _ _ _ _ _ w461]
        tunnel: w357 -> [_ w369 _ _ _ _ _ _ _ _ _]
        frame "ch-relay on", Default {
          n170 = case shown="0, Default" w360 {
            tunnel: [hw-control."Relay1" ("cmd") hw-control."Relay2" ("cmd") hw-control."Relay3" ("cmd") hw-control."Relay4" ("cmd") hw-control."Relay5" ("cmd") hw-control."Relay6" ("cmd")] -> w361
            frame 0, Default {
            }
            frame 1 {
            }
            frame 2 {
            }
            frame 3 {
            }
            frame 4 {
            }
            frame 5 {
            }
          }
          n171 = call "sub_hw-set.vi"("cmd"=w361, "onoff"=TRUE) -> ()  [unwired: 9 in, 1 out]
        }
        frame "hw set" {
          n172 = call "sub_hw-set.vi"("cmd"=hw-control."AO 0v") -> ("error out"=w370:errorcluster)  [unwired: 10 in]
          n173 = disable-structure shown="Disabled" {
            disable-tunnel: w370 -> [w374 _]
            disable-tunnel: w369 -> [w373 _]
            frame Disabled {
              n174 = case shown="1, Default" w373 {
                tunnel: w374 -> [w376 _]
                frame 0 {
                  n175 = call "sub_hw-set.vi"("cmd"=hw-control."DSP1500 set", "error in"=w376) -> ("error out"=w375:errorcluster)  [unwired: 9 in]
                  n176 = call "sub_hw-set.vi"("cmd"=hw-control."BP4610 set", "error in"=w375) -> ()  [unwired: 9 in, 1 out]
                }
                frame 1, Default {
                }
              }
            }
            frame Enabled {
            }
          }
          n177 = call "fgv_UI-set.vi"("cmd"=UI."DL950 graph clear") -> ()  [unwired: 10 in, 1 out]
        }
        frame "Pwr-in on" {
          n178 = call "fgv_time-check.vi"("cmd"=cmd_timecheck."pwr-in on start") -> ("error out"=w383:errorcluster)  [unwired: 9 in, 1 out]
          n179 = call "sub_hw-set.vi"("cmd"=hw-control."BP4610 onoff", "error in"=w383, "onoff"=TRUE) -> ("error out"=w382:errorcluster)  [unwired: 8 in]
          n180 = call "sub_hw-set.vi"("cmd"=hw-control."AO 12v", "error in"=w382) -> ("error out"=w381:errorcluster)  [unwired: 9 in]
          n181 = Wait (ms)(milliseconds to wait=u32 100) -> ()  [unwired: 1 out]
          n182 = call "Stall Data Flow.vim"("value in"=w381, "milliseconds to wait"=u32 500 ("dt")) -> ("value out"=w390:errorcluster)  [unwired: 1 out]
          n183 = call "fgv_time-check.vi"("cmd"=cmd_timecheck."NF read start", "error in (no error)"=w390) -> ("error out"=w389:errorcluster)  [unwired: 8 in, 1 out]
          n184 = for {
            N: 3 -> [_]
            shift-right: [w400] -> w387
            shift-left: w389 -> [w401]
            n185 = call "fgv_4610_visa.vi"("cmd"=BP4610_cmd."read", "error in"=w401) -> ("error out"=w400:errorcluster)  [unwired: 9 in]
          }
          n186 = call "fgv_time-check.vi"("cmd"=cmd_timecheck."NF read stop", "error in (no error)"=w387) -> ("error out"=w386:errorcluster)  [unwired: 8 in, 1 out]
          n187 = call "Stall Data Flow.vim"("value in"=w386, "milliseconds to wait"=u32 200 ("dt")) -> ("value out"=w380:errorcluster)  [unwired: 1 out]
          n188 = call "sub_hw-set.vi"("cmd"=hw-control."AO 0v", "error in"=w380) -> ("error out"=w379:errorcluster)  [unwired: 9 in]
          n189 = call "fgv_time-check.vi"("cmd"=cmd_timecheck."pwr-in on stop", "error in (no error)"=w379) -> ()  [unwired: 8 in, 2 out]
        }
        frame "Pwr-out on" {
          n190 = call "fgv_time-check.vi"("cmd"=cmd_timecheck."pwr-out on start") -> ("error out"=w405:errorcluster)  [unwired: 9 in, 1 out]
          n191 = call "sub_hw-set.vi"("cmd"=hw-control."DSP1500 onoff", "error in"=w405, "onoff"=TRUE) -> ("error out"=w408:errorcluster)  [unwired: 8 in]
          n192 = flat-sequence {
            tunnel: [w415] -> w409
            tunnel: w408 -> [w415]
            frame #0 {
              n193 = Wait (ms)(milliseconds to wait=u32 200) -> ()  [unwired: 1 out]
            }
          }
          n194 = call "sub_breakdown-check.vi"("breakdown type"=breakdown."output pwr", "error in (no error)"=w409) -> ("error out"=w407:errorcluster)  [unwired: 9 in]
          n195 = flat-sequence {
            tunnel: w407 -> [w413]
            tunnel: [w413] -> w403
            frame #0 {
              n196 = Wait (ms)(milliseconds to wait=u32 500) -> ()  [unwired: 1 out]
            }
          }
          n197 = call "fgv_time-check.vi"("cmd"=cmd_timecheck."pwr-out on stop", "error in (no error)"=w403) -> ()  [unwired: 8 in, 2 out]
        }
        frame "AO on" {
          n198 = call "offTimeCheck.vi"("cmd"=cmd_offtimecheck."check") -> ("error out"=w418:errorcluster)  [unwired: 10 in]
          n199 = call "sub_hw-set.vi"("cmd"=hw-control."AO wave", "error in"=w418, "onoff"=TRUE) -> ("error out"=w417:errorcluster)  [unwired: 8 in]
          n200 = call "offTimeCheck.vi"("error in (no error)"=w417, "cmd"=cmd_offtimecheck."start") -> ()  [unwired: 9 in, 1 out]
        }
        frame "AO 0v" {
          n201 = disable-structure shown="Disabled" {
            frame Disabled {
              n202 = call "sub_hw-set.vi"("cmd"=hw-control."AO 0v") -> ()  [unwired: 10 in, 1 out]
            }
            frame Enabled {
            }
          }
        }
        frame "Pwr-in off" {
          n203 = call "fgv_time-check.vi"("cmd"=cmd_timecheck."pwr-in off start") -> ("error out"=w426:errorcluster)  [unwired: 9 in, 1 out]
          n204 = call "sub_hw-set.vi"("cmd"=hw-control."BP4610 onoff", "error in"=w426, "onoff"=FALSE) -> ("error out"=w424:errorcluster)  [unwired: 8 in]
          n205 = call "fgv_time-check.vi"("cmd"=cmd_timecheck."pwr-in off start", "error in (no error)"=w424) -> ()  [unwired: 8 in, 2 out]
        }
        frame "Relay-all off" {
          n206 = call "fgv_time-check.vi"("cmd"=cmd_timecheck."relay-all off start") -> ("error out"=w432:errorcluster)  [unwired: 9 in, 1 out]
          n207 = call "sub_hw-set.vi"("cmd"=hw-control."relay all-off", "error in"=w432, "onoff"=FALSE) -> ("error out"=w430:errorcluster)  [unwired: 8 in]
          n208 = call "fgv_time-check.vi"("cmd"=cmd_timecheck."relay-all off stop", "error in (no error)"=w430) -> ()  [unwired: 8 in, 2 out]
        }
        frame "Pwr-out off" {
          n209 = call "fgv_time-check.vi"("cmd"=cmd_timecheck."pwr-out off start") -> ("error out"=w438:errorcluster)  [unwired: 9 in, 1 out]
          n210 = call "sub_hw-set.vi"("cmd"=hw-control."DSP1500 onoff", "error in"=w438, "onoff"=FALSE) -> ("error out"=w436:errorcluster)  [unwired: 8 in]
          n211 = call "fgv_time-check.vi"("cmd"=cmd_timecheck."pwr-out off stop", "error in (no error)"=w436) -> ()  [unwired: 8 in, 2 out]
        }
        frame "Discharge" {
          n212 = call "fgv_time-check.vi"("cmd"=cmd_timecheck."discharge start") -> ("error out"=w447:errorcluster)  [unwired: 9 in, 1 out]
          n213 = call "sub_hw-set.vi"("cmd"=hw-control."Discharge", "error in"=w447, "onoff"=TRUE) -> ("error out"=w446:errorcluster)  [unwired: 8 in]
          n214 = call "sub_hw-set.vi"("cmd"=hw-control."Discharge check", "error in"=w446) -> ("error out"=w445:errorcluster)  [unwired: 9 in]
          n215 = call "sub_hw-set.vi"("cmd"=hw-control."Discharge", "error in"=w445, "onoff"=FALSE) -> ("error out"=w442:errorcluster)  [unwired: 8 in]
          n216 = flat-sequence {
            tunnel: [w454] -> w443
            tunnel: w442 -> [w454]
            frame #0 {
              n217 = Wait (ms)(milliseconds to wait=u32 2000) -> ()  [unwired: 1 out]
            }
          }
          n218 = call "fgv_time-check.vi"("cmd"=cmd_timecheck."discharge stop", "error in (no error)"=w443) -> ()  [unwired: 8 in, 2 out]
        }
        frame "950 read" {
          n219 = call "fgv_time-check.vi"("cmd"=cmd_timecheck."950 read start") -> ("error out"=w458:errorcluster)  [unwired: 9 in, 1 out]
          n220 = call "sub_hw-set.vi"("cmd"=hw-control."DL950 read seq", "error in"=w458, "DUT Ch"=w461) -> ("error out"=w456:errorcluster)  [unwired: 8 in]
          n221 = call "fgv_time-check.vi"("cmd"=cmd_timecheck."950 read stop", "error in (no error)"=w456) -> ()  [unwired: 8 in, 2 out]
        }
      }
    }
    frame "B3" {
      n222 = case shown="\"AO on\"" w464 {
        tunnel: w465 -> [w466 _ _ _ _ _ _ _ _ _ w566]
        tunnel: w463 -> [_ w475 _ _ _ _ _ _ _ _ _]
        frame "ch-relay on", Default {
          n223 = case shown="0, Default" w466 {
            tunnel: [hw-control."Relay1" ("cmd") hw-control."Relay2" ("cmd") hw-control."Relay3" ("cmd") hw-control."Relay4" ("cmd") hw-control."Relay5" ("cmd") hw-control."Relay6" ("cmd")] -> w467
            frame 0, Default {
            }
            frame 1 {
            }
            frame 2 {
            }
            frame 3 {
            }
            frame 4 {
            }
            frame 5 {
            }
          }
          n224 = call "sub_hw-set.vi"("cmd"=w467, "onoff"=TRUE) -> ()  [unwired: 9 in, 1 out]
        }
        frame "hw set" {
          n225 = call "sub_hw-set.vi"("cmd"=hw-control."AO 0v") -> ("error out"=w476:errorcluster)  [unwired: 10 in]
          n226 = disable-structure shown="Enabled" {
            disable-tunnel: w476 -> [w480 _]
            disable-tunnel: w475 -> [w479 _]
            frame Disabled {
              n227 = case shown="1, Default" w479 {
                tunnel: w480 -> [w482 _]
                frame 0 {
                  n228 = call "sub_hw-set.vi"("cmd"=hw-control."DSP1500 set", "error in"=w482) -> ("error out"=w481:errorcluster)  [unwired: 9 in]
                  n229 = call "sub_hw-set.vi"("cmd"=hw-control."BP4610 set", "error in"=w481) -> ()  [unwired: 9 in, 1 out]
                }
                frame 1, Default {
                }
              }
            }
            frame Enabled {
            }
          }
          n230 = call "fgv_UI-set.vi"("cmd"=UI."DL950 graph clear") -> ()  [unwired: 10 in, 1 out]
        }
        frame "Pwr-in on" {
          n231 = call "fgv_time-check.vi"("cmd"=cmd_timecheck."pwr-in on start") -> ("error out"=w489:errorcluster)  [unwired: 9 in, 1 out]
          n232 = call "sub_hw-set.vi"("cmd"=hw-control."BP4610 onoff", "error in"=w489, "onoff"=TRUE) -> ("error out"=w488:errorcluster)  [unwired: 8 in]
          n233 = call "sub_hw-set.vi"("cmd"=hw-control."AO 12v", "error in"=w488) -> ("error out"=w487:errorcluster)  [unwired: 9 in]
          n234 = call "Stall Data Flow.vim"("value in"=w487, "milliseconds to wait"=u32 500 ("dt")) -> ("value out"=w496:errorcluster)  [unwired: 1 out]
          n235 = call "fgv_time-check.vi"("cmd"=cmd_timecheck."NF read start", "error in (no error)"=w496) -> ("error out"=w495:errorcluster)  [unwired: 8 in, 1 out]
          n236 = for {
            N: 3 -> [_]
            shift-right: [w505] -> w493
            shift-left: w495 -> [w506]
            n237 = call "fgv_4610_visa.vi"("cmd"=BP4610_cmd."read", "error in"=w506) -> ("error out"=w505:errorcluster)  [unwired: 9 in]
          }
          n238 = call "fgv_time-check.vi"("cmd"=cmd_timecheck."NF read stop", "error in (no error)"=w493) -> ("error out"=w492:errorcluster)  [unwired: 8 in, 1 out]
          n239 = call "Stall Data Flow.vim"("value in"=w492, "milliseconds to wait"=u32 200 ("dt")) -> ("value out"=w486:errorcluster)  [unwired: 1 out]
          n240 = call "sub_hw-set.vi"("cmd"=hw-control."AO 0v", "error in"=w486) -> ("error out"=w485:errorcluster)  [unwired: 9 in]
          n241 = call "fgv_time-check.vi"("cmd"=cmd_timecheck."pwr-in on stop", "error in (no error)"=w485) -> ()  [unwired: 8 in, 2 out]
        }
        frame "Pwr-out on" {
          n242 = call "fgv_time-check.vi"("cmd"=cmd_timecheck."pwr-out on start") -> ("error out"=w510:errorcluster)  [unwired: 9 in, 1 out]
          n243 = call "sub_hw-set.vi"("cmd"=hw-control."DSP1500 onoff", "error in"=w510, "onoff"=TRUE) -> ("error out"=w513:errorcluster)  [unwired: 8 in]
          n244 = flat-sequence {
            tunnel: [w520] -> w514
            tunnel: w513 -> [w520]
            frame #0 {
              n245 = Wait (ms)(milliseconds to wait=u32 200) -> ()  [unwired: 1 out]
            }
          }
          n246 = call "sub_breakdown-check.vi"("breakdown type"=breakdown."output pwr", "error in (no error)"=w514) -> ("error out"=w512:errorcluster)  [unwired: 9 in]
          n247 = flat-sequence {
            tunnel: w512 -> [w518]
            tunnel: [w518] -> w508
            frame #0 {
              n248 = Wait (ms)(milliseconds to wait=u32 500) -> ()  [unwired: 1 out]
            }
          }
          n249 = call "fgv_time-check.vi"("cmd"=cmd_timecheck."pwr-out on stop", "error in (no error)"=w508) -> ()  [unwired: 8 in, 2 out]
        }
        frame "AO on" {
          n250 = call "offTimeCheck.vi"("cmd"=cmd_offtimecheck."check") -> ("error out"=w523:errorcluster)  [unwired: 10 in]
          n251 = call "sub_hw-set.vi"("cmd"=hw-control."AO wave", "error in"=w523, "onoff"=TRUE) -> ("error out"=w522:errorcluster)  [unwired: 8 in]
          n252 = call "offTimeCheck.vi"("error in (no error)"=w522, "cmd"=cmd_offtimecheck."start") -> ()  [unwired: 9 in, 1 out]
        }
        frame "AO 0v" {
          n253 = disable-structure shown="Disabled" {
            frame Disabled {
              n254 = call "sub_hw-set.vi"("cmd"=hw-control."AO 0v") -> ()  [unwired: 10 in, 1 out]
            }
            frame Enabled {
            }
          }
        }
        frame "Pwr-in off" {
          n255 = call "fgv_time-check.vi"("cmd"=cmd_timecheck."pwr-in off start") -> ("error out"=w531:errorcluster)  [unwired: 9 in, 1 out]
          n256 = call "sub_hw-set.vi"("cmd"=hw-control."BP4610 onoff", "error in"=w531, "onoff"=FALSE) -> ("error out"=w529:errorcluster)  [unwired: 8 in]
          n257 = call "fgv_time-check.vi"("cmd"=cmd_timecheck."pwr-in off start", "error in (no error)"=w529) -> ()  [unwired: 8 in, 2 out]
        }
        frame "Relay-all off" {
          n258 = call "fgv_time-check.vi"("cmd"=cmd_timecheck."relay-all off start") -> ("error out"=w537:errorcluster)  [unwired: 9 in, 1 out]
          n259 = call "sub_hw-set.vi"("cmd"=hw-control."relay all-off", "error in"=w537, "onoff"=FALSE) -> ("error out"=w535:errorcluster)  [unwired: 8 in]
          n260 = call "fgv_time-check.vi"("cmd"=cmd_timecheck."relay-all off stop", "error in (no error)"=w535) -> ()  [unwired: 8 in, 2 out]
        }
        frame "Pwr-out off" {
          n261 = call "fgv_time-check.vi"("cmd"=cmd_timecheck."pwr-out off start") -> ("error out"=w543:errorcluster)  [unwired: 9 in, 1 out]
          n262 = call "sub_hw-set.vi"("cmd"=hw-control."DSP1500 onoff", "error in"=w543, "onoff"=FALSE) -> ("error out"=w541:errorcluster)  [unwired: 8 in]
          n263 = call "fgv_time-check.vi"("cmd"=cmd_timecheck."pwr-out off stop", "error in (no error)"=w541) -> ()  [unwired: 8 in, 2 out]
        }
        frame "Discharge" {
          n264 = call "fgv_time-check.vi"("cmd"=cmd_timecheck."discharge start") -> ("error out"=w552:errorcluster)  [unwired: 9 in, 1 out]
          n265 = call "sub_hw-set.vi"("cmd"=hw-control."Discharge", "error in"=w552, "onoff"=TRUE) -> ("error out"=w551:errorcluster)  [unwired: 8 in]
          n266 = call "sub_hw-set.vi"("cmd"=hw-control."Discharge check", "error in"=w551) -> ("error out"=w550:errorcluster)  [unwired: 9 in]
          n267 = call "sub_hw-set.vi"("cmd"=hw-control."Discharge", "error in"=w550, "onoff"=FALSE) -> ("error out"=w547:errorcluster)  [unwired: 8 in]
          n268 = flat-sequence {
            tunnel: [w559] -> w548
            tunnel: w547 -> [w559]
            frame #0 {
              n269 = Wait (ms)(milliseconds to wait=u32 2000) -> ()  [unwired: 1 out]
            }
          }
          n270 = call "fgv_time-check.vi"("cmd"=cmd_timecheck."discharge stop", "error in (no error)"=w548) -> ()  [unwired: 8 in, 2 out]
        }
        frame "950 read" {
          n271 = call "fgv_time-check.vi"("cmd"=cmd_timecheck."950 read start") -> ("error out"=w563:errorcluster)  [unwired: 9 in, 1 out]
          n272 = call "sub_hw-set.vi"("cmd"=hw-control."DL950 read seq", "error in"=w563, "DUT Ch"=w566) -> ("error out"=w561:errorcluster)  [unwired: 8 in]
          n273 = call "fgv_time-check.vi"("cmd"=cmd_timecheck."950 read stop", "error in (no error)"=w561) -> ()  [unwired: 8 in, 2 out]
        }
      }
    }
    frame "Oper_LV" {
      n274 = case shown="\"950 read\"" w569 {
        tunnel: w570 -> [w571 _ _ _ _ _ _ _ _ _ w675]
        tunnel: w568 -> [_ w580 _ _ _ _ _ _ _ _ _]
        frame "ch-relay on", Default {
          n275 = case shown="0, Default" w571 {
            tunnel: [hw-control."Relay1" ("cmd") hw-control."Relay2" ("cmd") hw-control."Relay3" ("cmd") hw-control."Relay4" ("cmd") hw-control."Relay5" ("cmd") hw-control."Relay6" ("cmd")] -> w572
            frame 0, Default {
            }
            frame 1 {
            }
            frame 2 {
            }
            frame 3 {
            }
            frame 4 {
            }
            frame 5 {
            }
          }
          n276 = call "sub_hw-set.vi"("cmd"=w572, "onoff"=TRUE) -> ()  [unwired: 9 in, 1 out]
        }
        frame "hw set" {
          n277 = call "sub_hw-set.vi"("cmd"=hw-control."AO 0v") -> ("error out"=w581:errorcluster)  [unwired: 10 in]
          n278 = disable-structure shown="Disabled" {
            disable-tunnel: w581 -> [w585 _]
            disable-tunnel: w580 -> [w584 _]
            frame Disabled {
              n279 = case shown="1, Default" w584 {
                tunnel: w585 -> [w587 _]
                frame 0 {
                  n280 = call "sub_hw-set.vi"("cmd"=hw-control."DSP1500 set", "error in"=w587) -> ("error out"=w586:errorcluster)  [unwired: 9 in]
                  n281 = call "sub_hw-set.vi"("cmd"=hw-control."BP4610 set", "error in"=w586) -> ()  [unwired: 9 in, 1 out]
                }
                frame 1, Default {
                }
              }
            }
            frame Enabled {
            }
          }
          n282 = call "fgv_UI-set.vi"("cmd"=UI."DL950 graph clear") -> ()  [unwired: 10 in, 1 out]
        }
        frame "Pwr-in on" {
          n283 = call "fgv_time-check.vi"("cmd"=cmd_timecheck."pwr-in on start") -> ("error out"=w594:errorcluster)  [unwired: 9 in, 1 out]
          n284 = call "sub_hw-set.vi"("cmd"=hw-control."BP4610 onoff", "error in"=w594, "onoff"=TRUE) -> ("error out"=w593:errorcluster)  [unwired: 8 in]
          n285 = call "sub_hw-set.vi"("cmd"=hw-control."AO 12v", "error in"=w593) -> ("error out"=w592:errorcluster)  [unwired: 9 in]
          n286 = call "Stall Data Flow.vim"("value in"=w592, "milliseconds to wait"=u32 100 ("dt")) -> ("value out"=w601:errorcluster)  [unwired: 1 out]
          n287 = call "fgv_time-check.vi"("cmd"=cmd_timecheck."NF read start", "error in (no error)"=w601) -> ("error out"=w600:errorcluster)  [unwired: 8 in, 1 out]
          n288 = for {
            N: 2 -> [_]
            shift-right: [w610] -> w598
            shift-left: w600 -> [w611]
            n289 = call "fgv_4610_visa.vi"("cmd"=BP4610_cmd."read", "error in"=w611) -> ("error out"=w610:errorcluster)  [unwired: 9 in]
          }
          n290 = call "fgv_time-check.vi"("cmd"=cmd_timecheck."NF read stop", "error in (no error)"=w598) -> ("error out"=w597:errorcluster)  [unwired: 8 in, 1 out]
          n291 = call "Stall Data Flow.vim"("value in"=w597, "milliseconds to wait"=u32 100 ("dt")) -> ("value out"=w591:errorcluster)  [unwired: 1 out]
          n292 = call "sub_hw-set.vi"("cmd"=hw-control."AO 0v", "error in"=w591) -> ("error out"=w590:errorcluster)  [unwired: 9 in]
          n293 = call "fgv_time-check.vi"("cmd"=cmd_timecheck."pwr-in on stop", "error in (no error)"=w590) -> ()  [unwired: 8 in, 2 out]
        }
        frame "Pwr-out on" {
          n294 = call "fgv_time-check.vi"("cmd"=cmd_timecheck."pwr-out on start") -> ("error out"=w618:errorcluster)  [unwired: 9 in, 1 out]
          n295 = call "sub_hw-set.vi"("cmd"=hw-control."DSP1500 onoff", "error in"=w618, "onoff"=TRUE) -> ("error out"=w621:errorcluster)  [unwired: 8 in]
          n296 = global read "Glob_Ref.vi" "simulation"() -> (w613:bool)
          n297 = call "Stall Data Flow.vim"("value in"=w621, "milliseconds to wait"=u32 100) -> ("value out"=w622:errorcluster)  [unwired: 1 out]
          n298 = case shown="True" w613 {
            tunnel: w622 -> [w625 w627]
            tunnel: [w625 w626] -> w620
            frame False {
            }
            frame True {
              n299 = call "sub_breakdown-check.vi"("breakdown type"=breakdown."output pwr", "error in (no error)"=w627) -> ("error out"=w626:errorcluster)  [unwired: 9 in]
            }
          }
          n300 = call "Stall Data Flow.vim"("value in"=w620, "milliseconds to wait"=u32 400) -> ("value out"=w616:errorcluster)  [unwired: 1 out]
          n301 = call "fgv_time-check.vi"("cmd"=cmd_timecheck."pwr-out on stop", "error in (no error)"=w616) -> ()  [unwired: 8 in, 2 out]
        }
        frame "AO on" {
          n302 = call "offTimeCheck.vi"("cmd"=cmd_offtimecheck."check") -> ("error out"=w630:errorcluster)  [unwired: 10 in]
          n303 = call "Trig_TimeCheck.vi"("error in (no error)"=w630, "cmd"=cmd_offtimecheck."start") -> ("error out"=w629:errorcluster)  [unwired: 9 in]
          n304 = call "sub_hw-set.vi"("cmd"=hw-control."AO wave", "error in"=w629, "onoff"=TRUE) -> ("error out"=w632:errorcluster)  [unwired: 8 in]
          n305 = call "offTimeCheck.vi"("error in (no error)"=w632, "cmd"=cmd_offtimecheck."start") -> ()  [unwired: 9 in, 1 out]
        }
        frame "AO 0v" {
          n306 = disable-structure shown="Disabled" {
            frame Disabled {
              n307 = call "sub_hw-set.vi"("cmd"=hw-control."AO 0v") -> ()  [unwired: 10 in, 1 out]
            }
            frame Enabled {
            }
          }
        }
        frame "Pwr-in off" {
          n308 = call "fgv_time-check.vi"("cmd"=cmd_timecheck."pwr-in off start") -> ("error out"=w640:errorcluster)  [unwired: 9 in, 1 out]
          n309 = call "sub_hw-set.vi"("cmd"=hw-control."BP4610 onoff", "error in"=w640, "onoff"=FALSE) -> ("error out"=w638:errorcluster)  [unwired: 8 in]
          n310 = call "fgv_time-check.vi"("cmd"=cmd_timecheck."pwr-in off start", "error in (no error)"=w638) -> ()  [unwired: 8 in, 2 out]
        }
        frame "Relay-all off" {
          n311 = call "fgv_time-check.vi"("cmd"=cmd_timecheck."relay-all off start") -> ("error out"=w646:errorcluster)  [unwired: 9 in, 1 out]
          n312 = call "sub_hw-set.vi"("cmd"=hw-control."relay all-off", "error in"=w646, "onoff"=FALSE) -> ("error out"=w644:errorcluster)  [unwired: 8 in]
          n313 = call "fgv_time-check.vi"("cmd"=cmd_timecheck."relay-all off stop", "error in (no error)"=w644) -> ()  [unwired: 8 in, 2 out]
        }
        frame "Pwr-out off" {
          n314 = call "fgv_time-check.vi"("cmd"=cmd_timecheck."pwr-out off start") -> ("error out"=w652:errorcluster)  [unwired: 9 in, 1 out]
          n315 = call "sub_hw-set.vi"("cmd"=hw-control."DSP1500 onoff", "error in"=w652, "onoff"=FALSE) -> ("error out"=w650:errorcluster)  [unwired: 8 in]
          n316 = call "fgv_time-check.vi"("cmd"=cmd_timecheck."pwr-out off stop", "error in (no error)"=w650) -> ()  [unwired: 8 in, 2 out]
        }
        frame "Discharge" {
          n317 = call "fgv_time-check.vi"("cmd"=cmd_timecheck."discharge start") -> ("error out"=w661:errorcluster)  [unwired: 9 in, 1 out]
          n318 = call "sub_hw-set.vi"("cmd"=hw-control."Discharge", "error in"=w661, "onoff"=TRUE) -> ("error out"=w660:errorcluster)  [unwired: 8 in]
          n319 = call "sub_hw-set.vi"("cmd"=hw-control."Discharge check", "error in"=w660) -> ("error out"=w659:errorcluster)  [unwired: 9 in]
          n320 = call "sub_hw-set.vi"("cmd"=hw-control."Discharge", "error in"=w659, "onoff"=FALSE) -> ("error out"=w656:errorcluster)  [unwired: 8 in]
          n321 = flat-sequence {
            tunnel: [w668] -> w657
            tunnel: w656 -> [w668]
            frame #0 {
              n322 = Wait (ms)(milliseconds to wait=u32 2000) -> ()  [unwired: 1 out]
            }
          }
          n323 = call "fgv_time-check.vi"("cmd"=cmd_timecheck."discharge stop", "error in (no error)"=w657) -> ()  [unwired: 8 in, 2 out]
        }
        frame "950 read" {
          n324 = call "fgv_time-check.vi"("cmd"=cmd_timecheck."950 read start") -> ("error out"=w672:errorcluster)  [unwired: 9 in, 1 out]
          n325 = call "sub_hw-set.vi"("cmd"=hw-control."DL950 read seq", "error in"=w672, "DUT Ch"=w675) -> ("error out"=w670:errorcluster)  [unwired: 8 in]
          n326 = call "fgv_time-check.vi"("cmd"=cmd_timecheck."950 read stop", "error in (no error)"=w670) -> ()  [unwired: 8 in, 2 out]
        }
      }
    }
    frame "Oper_HV" {
      n327 = case shown="\"Pwr-out on\"" w679 {
        tunnel: w677 -> [_ _ _ _ _ _ _ _ _ _ _]
        tunnel: w680 -> [w681 _ _ _ _ _ _ _ _ _ w783]
        tunnel: w678 -> [_ w690 _ _ _ _ _ _ _ _ _]
        frame "ch-relay on", Default {
          n328 = case shown="2" w681 {
            tunnel: [hw-control."Relay1" ("cmd") hw-control."Relay2" ("cmd") hw-control."Relay3" ("cmd") hw-control."Relay4" ("cmd") hw-control."Relay5" ("cmd") hw-control."Relay6" ("cmd")] -> w682
            frame 0, Default {
            }
            frame 1 {
            }
            frame 2 {
            }
            frame 3 {
            }
            frame 4 {
            }
            frame 5 {
            }
          }
          n329 = call "sub_hw-set.vi"("cmd"=w682, "onoff"=TRUE) -> ()  [unwired: 9 in, 1 out]
        }
        frame "hw set" {
          n330 = call "sub_hw-set.vi"("cmd"=hw-control."AO 0v") -> ("error out"=w691:errorcluster)  [unwired: 10 in]
          n331 = disable-structure shown="Disabled" {
            disable-tunnel: w691 -> [w695 _]
            disable-tunnel: w690 -> [w694 _]
            frame Disabled {
              n332 = case shown="1, Default" w694 {
                tunnel: w695 -> [w697 _]
                frame 0 {
                  n333 = call "sub_hw-set.vi"("cmd"=hw-control."DSP1500 set", "error in"=w697) -> ("error out"=w696:errorcluster)  [unwired: 9 in]
                  n334 = call "sub_hw-set.vi"("cmd"=hw-control."BP4610 set", "error in"=w696) -> ()  [unwired: 9 in, 1 out]
                }
                frame 1, Default {
                }
              }
              n335 = call "fgv_UI-set.vi"("cmd"=UI."DL950 graph clear") -> ()  [unwired: 10 in, 1 out]
            }
            frame Enabled {
            }
          }
        }
        frame "Pwr-in on" {
          n336 = call "fgv_time-check.vi"("cmd"=cmd_timecheck."pwr-in on start") -> ("error out"=w704:errorcluster)  [unwired: 9 in, 1 out]
          n337 = call "sub_hw-set.vi"("cmd"=hw-control."BP4610 onoff", "error in"=w704, "onoff"=TRUE) -> ("error out"=w703:errorcluster)  [unwired: 8 in]
          n338 = call "sub_hw-set.vi"("cmd"=hw-control."AO 12v", "error in"=w703) -> ("error out"=w702:errorcluster)  [unwired: 9 in]
          n339 = call "Stall Data Flow.vim"("value in"=w702, "milliseconds to wait"=u32 50 ("dt")) -> ("value out"=w711:errorcluster)  [unwired: 1 out]
          n340 = call "fgv_time-check.vi"("cmd"=cmd_timecheck."NF read start", "error in (no error)"=w711) -> ("error out"=w710:errorcluster)  [unwired: 8 in, 1 out]
          n341 = for {
            N: 2 -> [_]
            shift-right: [w720] -> w708
            shift-left: w710 -> [w721]
            n342 = call "fgv_4610_visa.vi"("cmd"=BP4610_cmd."read", "error in"=w721) -> ("error out"=w720:errorcluster)  [unwired: 9 in]
          }
          n343 = call "fgv_time-check.vi"("cmd"=cmd_timecheck."NF read stop", "error in (no error)"=w708) -> ("error out"=w707:errorcluster)  [unwired: 8 in, 1 out]
          n344 = call "Stall Data Flow.vim"("value in"=w707, "milliseconds to wait"=u32 100 ("dt")) -> ("value out"=w701:errorcluster)  [unwired: 1 out]
          n345 = call "sub_hw-set.vi"("cmd"=hw-control."AO 0v", "error in"=w701) -> ("error out"=w700:errorcluster)  [unwired: 9 in]
          n346 = call "fgv_time-check.vi"("cmd"=cmd_timecheck."pwr-in on stop", "error in (no error)"=w700) -> ()  [unwired: 8 in, 2 out]
        }
        frame "Pwr-out on" {
          n347 = call "fgv_time-check.vi"("cmd"=cmd_timecheck."pwr-out on start") -> ("error out"=w725:errorcluster)  [unwired: 9 in, 1 out]
          n348 = call "sub_hw-set.vi"("cmd"=hw-control."DSP1500 onoff", "error in"=w725, "onoff"=TRUE) -> ("error out"=w728:errorcluster)  [unwired: 8 in]
          n349 = flat-sequence {
            tunnel: [w735] -> w729
            tunnel: w728 -> [w735]
            frame #0 {
              n350 = Wait (ms)(milliseconds to wait=u32 100) -> ()  [unwired: 1 out]
            }
          }
          n351 = call "sub_breakdown-check.vi"("breakdown type"=breakdown."output pwr", "error in (no error)"=w729) -> ("error out"=w727:errorcluster)  [unwired: 9 in]
          n352 = flat-sequence {
            tunnel: w727 -> [w733]
            tunnel: [w733] -> w723
            frame #0 {
              n353 = Wait (ms)(milliseconds to wait=u32 300) -> ()  [unwired: 1 out]
            }
          }
          n354 = call "fgv_time-check.vi"("cmd"=cmd_timecheck."pwr-out on stop", "error in (no error)"=w723) -> ()  [unwired: 8 in, 2 out]
        }
        frame "AO on" {
          n355 = call "offTimeCheck.vi"("cmd"=cmd_offtimecheck."check") -> ("error out"=w738:errorcluster)  [unwired: 10 in]
          n356 = call "Trig_TimeCheck.vi"("error in (no error)"=w738, "cmd"=cmd_offtimecheck."start") -> ("error out"=w737:errorcluster)  [unwired: 9 in]
          n357 = call "sub_hw-set.vi"("cmd"=hw-control."AO wave", "error in"=w737, "onoff"=TRUE) -> ("error out"=w740:errorcluster)  [unwired: 8 in]
          n358 = call "offTimeCheck.vi"("error in (no error)"=w740, "cmd"=cmd_offtimecheck."start") -> ()  [unwired: 9 in, 1 out]
        }
        frame "AO 0v" {
          n359 = disable-structure shown="Disabled" {
            frame Disabled {
              n360 = call "sub_hw-set.vi"("cmd"=hw-control."AO 0v") -> ()  [unwired: 10 in, 1 out]
            }
            frame Enabled {
            }
          }
        }
        frame "Pwr-in off" {
          n361 = call "fgv_time-check.vi"("cmd"=cmd_timecheck."pwr-in off start") -> ("error out"=w748:errorcluster)  [unwired: 9 in, 1 out]
          n362 = call "sub_hw-set.vi"("cmd"=hw-control."BP4610 onoff", "error in"=w748, "onoff"=FALSE) -> ("error out"=w746:errorcluster)  [unwired: 8 in]
          n363 = call "fgv_time-check.vi"("cmd"=cmd_timecheck."pwr-in off start", "error in (no error)"=w746) -> ()  [unwired: 8 in, 2 out]
        }
        frame "Relay-all off" {
          n364 = call "fgv_time-check.vi"("cmd"=cmd_timecheck."relay-all off start") -> ("error out"=w754:errorcluster)  [unwired: 9 in, 1 out]
          n365 = call "sub_hw-set.vi"("cmd"=hw-control."relay all-off", "error in"=w754, "onoff"=FALSE) -> ("error out"=w752:errorcluster)  [unwired: 8 in]
          n366 = call "fgv_time-check.vi"("cmd"=cmd_timecheck."relay-all off stop", "error in (no error)"=w752) -> ()  [unwired: 8 in, 2 out]
        }
        frame "Pwr-out off" {
          n367 = call "fgv_time-check.vi"("cmd"=cmd_timecheck."pwr-out off start") -> ("error out"=w760:errorcluster)  [unwired: 9 in, 1 out]
          n368 = call "sub_hw-set.vi"("cmd"=hw-control."DSP1500 onoff", "error in"=w760, "onoff"=FALSE) -> ("error out"=w758:errorcluster)  [unwired: 8 in]
          n369 = call "fgv_time-check.vi"("cmd"=cmd_timecheck."pwr-out off stop", "error in (no error)"=w758) -> ()  [unwired: 8 in, 2 out]
        }
        frame "Discharge" {
          n370 = call "fgv_time-check.vi"("cmd"=cmd_timecheck."discharge start") -> ("error out"=w769:errorcluster)  [unwired: 9 in, 1 out]
          n371 = call "sub_hw-set.vi"("cmd"=hw-control."Discharge", "error in"=w769, "onoff"=TRUE) -> ("error out"=w768:errorcluster)  [unwired: 8 in]
          n372 = call "sub_hw-set.vi"("cmd"=hw-control."Discharge check", "error in"=w768) -> ("error out"=w767:errorcluster)  [unwired: 9 in]
          n373 = call "sub_hw-set.vi"("cmd"=hw-control."Discharge", "error in"=w767, "onoff"=FALSE) -> ("error out"=w764:errorcluster)  [unwired: 8 in]
          n374 = flat-sequence {
            tunnel: [w776] -> w765
            tunnel: w764 -> [w776]
            frame #0 {
              n375 = disable-structure shown="Disabled" {
                frame Disabled {
                  n376 = Wait (ms)(milliseconds to wait=u32 2000) -> ()  [unwired: 1 out]
                }
                frame Enabled {
                }
              }
            }
          }
          n377 = call "fgv_time-check.vi"("cmd"=cmd_timecheck."discharge stop", "error in (no error)"=w765) -> ()  [unwired: 8 in, 2 out]
        }
        frame "950 read" {
          n378 = call "fgv_time-check.vi"("cmd"=cmd_timecheck."950 read start") -> ("error out"=w780:errorcluster)  [unwired: 9 in, 1 out]
          n379 = call "sub_hw-set.vi"("cmd"=hw-control."DL950 read seq", "error in"=w780, "DUT Ch"=w783) -> ("error out"=w778:errorcluster)  [unwired: 8 in]
          n380 = call "fgv_time-check.vi"("cmd"=cmd_timecheck."950 read stop", "error in (no error)"=w778) -> ()  [unwired: 8 in, 2 out]
        }
      }
    }
    frame "ContR_LV" {
      n381 = case shown="\"950 read\"" w786 {
        tunnel: w787 -> [w788 _ _ _ _ _ _ _ _ _ w890]
        tunnel: w785 -> [_ w797 _ _ _ _ _ _ _ _ _]
        frame "ch-relay on", Default {
          n382 = case shown="0, Default" w788 {
            tunnel: [hw-control."Relay1" ("cmd") hw-control."Relay2" ("cmd") hw-control."Relay3" ("cmd") hw-control."Relay4" ("cmd") hw-control."Relay5" ("cmd") hw-control."Relay6" ("cmd")] -> w789
            frame 0, Default {
            }
            frame 1 {
            }
            frame 2 {
            }
            frame 3 {
            }
            frame 4 {
            }
            frame 5 {
            }
          }
          n383 = call "sub_hw-set.vi"("cmd"=w789, "onoff"=TRUE) -> ()  [unwired: 9 in, 1 out]
        }
        frame "hw set" {
          n384 = call "sub_hw-set.vi"("cmd"=hw-control."AO 0v") -> ("error out"=w798:errorcluster)  [unwired: 10 in]
          n385 = disable-structure shown="Enabled" {
            disable-tunnel: w798 -> [w802 _]
            disable-tunnel: w797 -> [w801 _]
            frame Disabled {
              n386 = case shown="1, Default" w801 {
                tunnel: w802 -> [w804 _]
                frame 0 {
                  n387 = call "sub_hw-set.vi"("cmd"=hw-control."DSP1500 set", "error in"=w804) -> ("error out"=w803:errorcluster)  [unwired: 9 in]
                  n388 = call "sub_hw-set.vi"("cmd"=hw-control."BP4610 set", "error in"=w803) -> ()  [unwired: 9 in, 1 out]
                }
                frame 1, Default {
                }
              }
            }
            frame Enabled {
            }
          }
          n389 = call "fgv_UI-set.vi"("cmd"=UI."DL950 graph clear") -> ()  [unwired: 10 in, 1 out]
        }
        frame "Pwr-in on" {
          n390 = call "fgv_time-check.vi"("cmd"=cmd_timecheck."pwr-in on start") -> ("error out"=w811:errorcluster)  [unwired: 9 in, 1 out]
          n391 = call "sub_hw-set.vi"("cmd"=hw-control."BP4610 onoff", "error in"=w811, "onoff"=TRUE) -> ("error out"=w810:errorcluster)  [unwired: 8 in]
          n392 = call "sub_hw-set.vi"("cmd"=hw-control."AO 12v", "error in"=w810) -> ("error out"=w809:errorcluster)  [unwired: 9 in]
          n393 = call "Stall Data Flow.vim"("value in"=w809, "milliseconds to wait"=u32 100 ("dt")) -> ("value out"=w818:errorcluster)  [unwired: 1 out]
          n394 = call "fgv_time-check.vi"("cmd"=cmd_timecheck."NF read start", "error in (no error)"=w818) -> ("error out"=w817:errorcluster)  [unwired: 8 in, 1 out]
          n395 = for {
            N: 2 -> [_]
            shift-right: [w827] -> w815
            shift-left: w817 -> [w828]
            n396 = call "fgv_4610_visa.vi"("cmd"=BP4610_cmd."read", "error in"=w828) -> ("error out"=w827:errorcluster)  [unwired: 9 in]
          }
          n397 = call "fgv_time-check.vi"("cmd"=cmd_timecheck."NF read stop", "error in (no error)"=w815) -> ("error out"=w814:errorcluster)  [unwired: 8 in, 1 out]
          n398 = call "Stall Data Flow.vim"("value in"=w814, "milliseconds to wait"=u32 100 ("dt")) -> ("value out"=w808:errorcluster)  [unwired: 1 out]
          n399 = call "sub_hw-set.vi"("cmd"=hw-control."AO 0v", "error in"=w808) -> ("error out"=w807:errorcluster)  [unwired: 9 in]
          n400 = call "fgv_time-check.vi"("cmd"=cmd_timecheck."pwr-in on stop", "error in (no error)"=w807) -> ()  [unwired: 8 in, 2 out]
        }
        frame "Pwr-out on" {
          n401 = call "fgv_time-check.vi"("cmd"=cmd_timecheck."pwr-out on start") -> ("error out"=w832:errorcluster)  [unwired: 9 in, 1 out]
          n402 = call "sub_hw-set.vi"("cmd"=hw-control."DSP1500 onoff", "error in"=w832, "onoff"=TRUE) -> ("error out"=w835:errorcluster)  [unwired: 8 in]
          n403 = flat-sequence {
            tunnel: [w842] -> w836
            tunnel: w835 -> [w842]
            frame #0 {
              n404 = Wait (ms)(milliseconds to wait=u32 50) -> ()  [unwired: 1 out]
            }
          }
          n405 = call "sub_breakdown-check.vi"("breakdown type"=breakdown."output pwr", "error in (no error)"=w836) -> ("error out"=w834:errorcluster)  [unwired: 9 in]
          n406 = flat-sequence {
            tunnel: w834 -> [w840]
            tunnel: [w840] -> w830
            frame #0 {
              n407 = Wait (ms)(milliseconds to wait=u32 300) -> ()  [unwired: 1 out]
            }
          }
          n408 = call "fgv_time-check.vi"("cmd"=cmd_timecheck."pwr-out on stop", "error in (no error)"=w830) -> ()  [unwired: 8 in, 2 out]
        }
        frame "AO on" {
          n409 = call "offTimeCheck.vi"("cmd"=cmd_offtimecheck."check") -> ("error out"=w845:errorcluster)  [unwired: 10 in]
          n410 = call "Trig_TimeCheck.vi"("error in (no error)"=w845, "cmd"=cmd_offtimecheck."start") -> ("error out"=w844:errorcluster)  [unwired: 9 in]
          n411 = call "sub_hw-set.vi"("cmd"=hw-control."AO wave", "error in"=w844, "onoff"=TRUE) -> ("error out"=w847:errorcluster)  [unwired: 8 in]
          n412 = call "offTimeCheck.vi"("error in (no error)"=w847, "cmd"=cmd_offtimecheck."start") -> ()  [unwired: 9 in, 1 out]
        }
        frame "AO 0v" {
          n413 = disable-structure shown="Disabled" {
            frame Disabled {
              n414 = call "sub_hw-set.vi"("cmd"=hw-control."AO 0v") -> ()  [unwired: 10 in, 1 out]
            }
            frame Enabled {
            }
          }
        }
        frame "Pwr-in off" {
          n415 = call "fgv_time-check.vi"("cmd"=cmd_timecheck."pwr-in off start") -> ("error out"=w855:errorcluster)  [unwired: 9 in, 1 out]
          n416 = call "sub_hw-set.vi"("cmd"=hw-control."BP4610 onoff", "error in"=w855, "onoff"=FALSE) -> ("error out"=w853:errorcluster)  [unwired: 8 in]
          n417 = call "fgv_time-check.vi"("cmd"=cmd_timecheck."pwr-in off start", "error in (no error)"=w853) -> ()  [unwired: 8 in, 2 out]
        }
        frame "Relay-all off" {
          n418 = call "fgv_time-check.vi"("cmd"=cmd_timecheck."relay-all off start") -> ("error out"=w861:errorcluster)  [unwired: 9 in, 1 out]
          n419 = call "sub_hw-set.vi"("cmd"=hw-control."relay all-off", "error in"=w861, "onoff"=FALSE) -> ("error out"=w859:errorcluster)  [unwired: 8 in]
          n420 = call "fgv_time-check.vi"("cmd"=cmd_timecheck."relay-all off stop", "error in (no error)"=w859) -> ()  [unwired: 8 in, 2 out]
        }
        frame "Pwr-out off" {
          n421 = call "fgv_time-check.vi"("cmd"=cmd_timecheck."pwr-out off start") -> ("error out"=w867:errorcluster)  [unwired: 9 in, 1 out]
          n422 = call "sub_hw-set.vi"("cmd"=hw-control."DSP1500 onoff", "error in"=w867, "onoff"=FALSE) -> ("error out"=w865:errorcluster)  [unwired: 8 in]
          n423 = call "fgv_time-check.vi"("cmd"=cmd_timecheck."pwr-out off stop", "error in (no error)"=w865) -> ()  [unwired: 8 in, 2 out]
        }
        frame "Discharge" {
          n424 = call "fgv_time-check.vi"("cmd"=cmd_timecheck."discharge start") -> ("error out"=w876:errorcluster)  [unwired: 9 in, 1 out]
          n425 = call "sub_hw-set.vi"("cmd"=hw-control."Discharge", "error in"=w876, "onoff"=TRUE) -> ("error out"=w875:errorcluster)  [unwired: 8 in]
          n426 = call "sub_hw-set.vi"("cmd"=hw-control."Discharge check", "error in"=w875) -> ("error out"=w874:errorcluster)  [unwired: 9 in]
          n427 = call "sub_hw-set.vi"("cmd"=hw-control."Discharge", "error in"=w874, "onoff"=FALSE) -> ("error out"=w871:errorcluster)  [unwired: 8 in]
          n428 = flat-sequence {
            tunnel: [w883] -> w872
            tunnel: w871 -> [w883]
            frame #0 {
              n429 = Wait (ms)(milliseconds to wait=u32 2000) -> ()  [unwired: 1 out]
            }
          }
          n430 = call "fgv_time-check.vi"("cmd"=cmd_timecheck."discharge stop", "error in (no error)"=w872) -> ()  [unwired: 8 in, 2 out]
        }
        frame "950 read" {
          n431 = call "fgv_time-check.vi"("cmd"=cmd_timecheck."950 read start") -> ("error out"=w887:errorcluster)  [unwired: 9 in, 1 out]
          n432 = call "sub_hw-set.vi"("cmd"=hw-control."DL950 read seq", "error in"=w887, "DUT Ch"=w890) -> ("error out"=w885:errorcluster)  [unwired: 8 in]
          n433 = call "fgv_time-check.vi"("cmd"=cmd_timecheck."950 read stop", "error in (no error)"=w885) -> ()  [unwired: 8 in, 2 out]
        }
      }
    }
  }
  n434 = call "fgv_error.vi"("cmd"=rw."read", "error in (no error)"=w9) -> ("error out"=w4:errorcluster, "error cluster 2"=w8:T15)  [unwired: 8 in]
  n435 = Cluster To Array(cluster=w8) -> (array=w7:bool[])
  n436 = Or Array Elements(Boolean array=w7) -> (logical OR=w6:bool)
  n437 = case shown="True" w6 {
    tunnel: [w891 w893] -> w5
    tunnel: w4 -> [w891 w892]
    frame False {
    }
    frame True {
      n438 = call "fgv_stop_local.vi"("cmd"=init-r-stop."stop", "error in (no error)"=w892) -> ("error out"=w893:errorcluster)  [unwired: 8 in, 1 out]
    }
  }
  "error out" <- w5
